vi "UHR-Fleezers Control (fpga) - 11.0.vi"() -> ()   [LabVIEW 2012]
doc: "UHR-Fleezers Instrument Control Code (fpga)"
uses:
  <vilib>/Platform/TimedLoop/XDataNode/timing_clust.ctl
  <vilib>/Platform/TimedLoop/XDataNode/nitl_modes.ctl
  <vilib>/Platform/TimedLoop/XDataNode/wakeup.ctl
  <vilib>/rvi/eio/common/nirviEmuTemplateMethod_errors.vi
  <vilib>/rvi/interface/RandomDataEmulation/nirviRandomDataFPGAFIFO.vi
  <vilib>/rvi/interface/RandomDataEmulation/niFpgaRandomDataHandleErrors.vi
  <vilib>/rvi/Emulation/niFpgaSctlEmulationGetInTimedLoop.vi
  <vilib>/rvi/Emulation/niFpgaSctlEmulationGlobalWrite.vi
  <vilib>/rvi/Emulation/niFpgaSctlEmulationRegisterWithScheduler.vi
  <vilib>/rvi/Emulation/niFpgaSctlEmulationScheduler.vi
  <vilib>/Platform/TimedLoop/XDataNode/XDataNode.xnode
  <vilib>/eio/EIOMethodNode/EIOMethodNode.xnode
  <vilib>/eio/EIONode/EIONode.xnode
  <vilib>/rvi/DataTransferAndStorage/Container/XNode/niFpgaContainer.xnode
  <vilib>/rvi/interface/RandomDataEmulation/nirviRandomDataFpgaReadWriteTemplate.vi
  <vilib>/addons/control/pid/fpga.llb/XNode/niFpgaPID.xnode
  <vilib>/Platform/TimedLoop/XDataNode/XDNodeRunTimeDep.lvlib
panel:
  in  "Connector0/AO6":i16
  in  "Tab Control":T1(tab)=enum."Force FB"
  in  "Trap Pos to FIFO":bool
  in  "AI1 Sets to FIFO":T2={"Set 1"=TRUE, "Set 2"=TRUE, "Set 3"=FALSE}
  in  "N of AI1 Int Acq Sets":i16=2 min=1 max=3 step=1
  out "AI Late Counter":u16
  in  "ai count":u32=400
  out "AI late?":bool
  in  "+ phase":bool
  in  "Phase count adjustment":i16
  out "Relative phase":i16
  in  "AI to FIFO":bool
  out "BD1 Frequency Out 1":u64
  out "BD1 Frequency Out 2":u64
  out "Trap Pos FIFO Timeout":u16
  out "Trap AI FIFO Timeout":u16
  in  "Trap FIFO Set Timeout":i32
  in  "Tab Control 2":T3(tab)
  in  "Swap F1 and F2":bool
  in  "Freq or Amp switch first":bool=TRUE
  in  "Cont. Scan":bool
  in  "Abort scan":bool
  in  "Cycles per step":u64
  in  "Scan BD":bool
  in  "Number of scans":u16
  in  "Scan steps":u64
  in  "Scan freq.  increment":i64
  out "Scanning":bool
  in  "Start scan":bool
  in  "OSK Bd 1":bool
  in  "Reset Bd 1":bool
  in  "RD":bool
  in  "PMODE":bool
  in  "Direct RF Box \nCommunication":bool
  in  "Data BD 2":u8 format="%08b"
  in  "Data BD 1":u8 format="%08b"
  in  "Address":u8 format="%02x"
  in  "Update Data":bool
  in  "FPGA Controls\n RF Box":bool
  in  "Number Interlace Cycles":u8=2 min=1 max=3
  in  "Interlace Off Parameters":u8=1 min=1 max=3
  in  "Interlace ON/OFF":bool
  out "DIO Relative phase":i16
  in  "Phase count adjustment (DIO)":i16
  in  "+ phase (DIO)":bool
  out "DIO Late Counter":u16
  out "DIO Late?":bool
  in  "DIO count 1 (ticks)":u32=400
  in  "DIO count 2 (ticks)":u32=400
  in  "DIO count 3 (ticks)":u32=400
  out "AI2 Y Sum Set 2":i16
  out "AI2 Y Sum Set 1":i16
  in  "FB Gains Set 1":T4={"proportional gain (Kc)"=10, "integral gain (Kc*Ts/Ti)"=5, "derivative gain (Kc*Td/Ts)"=0}
  in  "FB Setpoint Set 1":i16 min=0 step=1
  in  "FB Reset Set 1":bool
  in  "FB On/Off Set 1":bool
  in  "FB Reset Set 2":bool
  in  "FB On/Off Set 2":bool
  in  "FB Setpoint Set 2":i16 min=0 step=1
  in  "FB Gains Set 2":T4={"proportional gain (Kc)"=10, "integral gain (Kc*Ts/Ti)"=5, "derivative gain (Kc*Td/Ts)"=0}
  in  "FB output range 2":cluster{"output high":i16, "output low":i16}={"output high"=3000, "output low"=0}
  in  "FB output range 1":cluster{"output high":i16, "output low":i16}={"output high"=3000, "output low"=0}
  out "Scan I":u64
  in  "Amp switch delay":u16=5
  in  "Freq switch delay":u16
  in  "BD 2 Amplitude 1":u16
  in  "BD 1 Amplitude 1":u16
  in  "BD 2 Frequency 1":u64
  in  "BD 1 Frequency 1":u64
  in  "BD 2 Amplitude 2":u16
  in  "BD 1 Amplitude 2":u16
  in  "BD 2 Frequency 2":u64
  in  "BD 1 Frequency 2":u64
  in  "BD 2 Amplitude 3":u16
  in  "BD 1 Amplitude 3":u16
  in  "BD 2 Frequency 3":u64
  in  "BD 1 Frequency 3":u64
  in  "Negate Diff?":bool
  in  "Diff FB Measurement?":bool
  in  "FB Trig Integrate":u32=1
  out "TTrig?":bool
  in  "TTrig Negate Pos":bool=TRUE
  out "Trap Pos FB Int Signal":fxp<+/-,24,9> format="%.18g"
  out "Trap Pos FB Int-Norm Signal":fxp<+/-,16,1> format="%.16g"
  in  "FPGA TTrig Thresh":i64
  in  "FPGA Trap Trig":bool
  out "Trap Pos FB Action":i64
  in  "Trap Pos. FB Offset Factor":i64
  in  "Trap Pos. FB Mult Factor":i64=2
  in  "Trap Pos. FB Range":T5={"output high"=0.999969482421875, "output low"=-1.0}
  in  "Trap Pos. FB Gains":T6={"proportional gain (Kc)"=0.0, "integral gain (Kc*Ts/Ti)"=10.0, "derivative gain (Kc*Td/Ts)"=0.0} {"proportional gain (Kc)" format="%.11g"; "integral gain (Kc*Ts/Ti)" format="%.11g"; "derivative gain (Kc*Td/Ts)" format="%.11g"}
  in  "Trap Pos. FB Reset":bool
  in  "Trap Pos FB Monitor T1 or T2":bool
  in  "AI1 X Scale":u16
  in  "Trap Pos FB Int Count":u16=100
  in  "Trap Pos FB Negate Action":bool
  out "AI1 X Set 2":fxp<+/-,16,1>
  out "AI1 X Set 1":fxp<+/-,16,1>
  in  "Trap Pos. FB SP":fxp<+/-,16,1>
  in  "Force feedback":bool
  out "TTrig Sig":i64
  out "TTrig Fin Thresh":i64
  out "Numeric":i32
  out "AO2 2":i16
  out "AO1 2":i16
  in  "1D or 2D Scan?":bool
  in  "Abort scan (MCL)":bool
  in  "MCL Scan Axis":bool
  in  "Cont. Scan (MCL)":bool
  out "Scan I (MCL)":u64
  in  "Number of scans (MCL)":u16
  out "Scanning MCL":bool
  in  "Scan steps (MCL)":u64
  in  "Cycles per step (MCL)":u64
  in  "Scan freq.  increment (MCL)":i16
  in  "Start scan (MCL)":bool
  in  "AO2":i16
  in  "AO1":i16
  out "MCL Late Counter":u16
  out "MCL Late?":bool
  in  "MCL count":u32=800
  out "MCL Relative Phase":i16
  in  "Phase count adjustment (MCL)":i16
  in  "+ phase (MCL)":bool
  in  "APD Gate Operating Mode":u8 max=2 step=1
  in  "Invert APD Gate":bool
  in  "APD Gate OFF Count":u32=100
  in  "APD Gate ON Count":u32=300
  out "APD 1 Gate Late Counter":u16
  out "APD 1 Gate Late?":bool
  out "APD 1 Gate Relative Phase":i16
  in  "Phase count adjustment (APD 1 Gate)":i16
  in  "+ phase (APD 1 Gate)":bool
  out "APD 2 Counts 0":u32
  out "APD 2 Counts 1":u32
  out "APD 1 Counts 0":u32
  out "APD 1 Counts 1":u32
  out "APD1 out state":bool
  in  "APD 2 AO scale factor":i16=1
  in  "APD 1 AO scale factor":i16=1
  in  "APD to FIFO":bool
  in  "APD Acq Rate Count":u32=20000000
  out "APD Acq Late Counter":u16
  out "APD Acq Late?":bool
  out "APD Acq Relative Phase":i16
  in  "Phase Count Adjustment (APD Acq)":i16
  in  "+ phase (APD Acq)":bool
  in  "Phase count adjustment (APD 2 Gate)":i16
  out "APD 2 Gate Late Counter":u16
  out "APD 2 Gate Late?":bool
  out "APD 2 Gate Relative Phase":i16
  in  "+ phase (APD 2 Gate)":bool
  out "APD2 out state":bool
  in  "Green Filter Flipper":bool
  in  "Green FB Count":u32=1200
  out "Green Late Counter":u16
  out "Green FB Late?":bool
  out "Green FB Relative Phase":i16
  in  "Phase count adjustment (Green FB)":i16=10
  in  "+ phase (Green FB)":bool
  out "Green FB Sum":i16
  in  "Green int current ON count adj":u32=150
  in  "Current Out":u16=30000
  in  "Green FB On/Off":bool
  in  "Green FB Setpoint":i16=250 min=0 step=1
  in  "Green FB Gains":T4={"proportional gain (Kc)"=10, "integral gain (Kc*Ts/Ti)"=5, "derivative gain (Kc*Td/Ts)"=0}
  in  "Green FB Reset":bool
  in  "Operating Mode 2":u8=2 max=2 step=1
  in  "Invert GI 2":bool
  in  "Green interlace OFF count 2":u32=900
  in  "Green interlace ON count 2":u32=300
  out "GI Late Counter 2":u16
  out "GI Late? 2":bool
  out "GI Relative phase 2":i16
  in  "Phase count adjustment (GI) 2":i16=20
  in  "+ phase (GI) 2":bool
  in  "Green interlace OFF count":u32=100
  out "GI Relative phase":i16
  in  "Phase count adjustment (GI)":i16
  in  "+ phase (GI)":bool
  out "GI Late?":bool
  in  "Green interlace ON count":u32=300
  out "GI Late Counter":u16
  in  "Invert GI":bool
  in  "Operating Mode":u8 max=2 step=1
  in  "+ phase (RI)":bool
  out "RI Relative phase":i16
  out "RI Late?":bool
  out "RI Late Counter":u16
  in  "Red interlace ON count":u32=300
  in  "Red interlace OFF count":u32=100
  in  "Invert RI":bool
  in  "Red Laser Operating Mode":u8 max=2 step=1
  in  "Phase count adjustment (RI)":i16
  out "Red FB Intensity":i16
  in  "Phase count adjustment (Red FB)":i16=10
  in  "Red FB Count":u32=1200
  out "Red Late Counter":u16
  out "Red FB Late?":bool
  out "Red FB Relative Phase":i16
  in  "+ phase (Red FB)":bool
  in  "Chassis2/Mod4/AO1":u16
  # "Only one of these can be on\nat a time:"
  # "Raster Scan AOD"
  # "1 (X)"
  # "2 (Y)"
  # "IR Intensity Feedback (RF BD 1)"
  # "FB Triggering Excitation Laser"
  # "AO1 (Y)"
  # "2D"
  # "1D"
  # "AO2 (X)"
  # "APD AO for aligning"
  # "Detection Loop"
  # "Green fluorescent laser digital gate interlacing loop"
  # "0 Forced ON\n1 Forced OFF\n2 Interlacing"
  # "Red fluorescent laser digital gate interlacing loop"
  # "Detection Loop"
  # "0 Forced ON\n1 Forced OFF\n2 Interlacing"
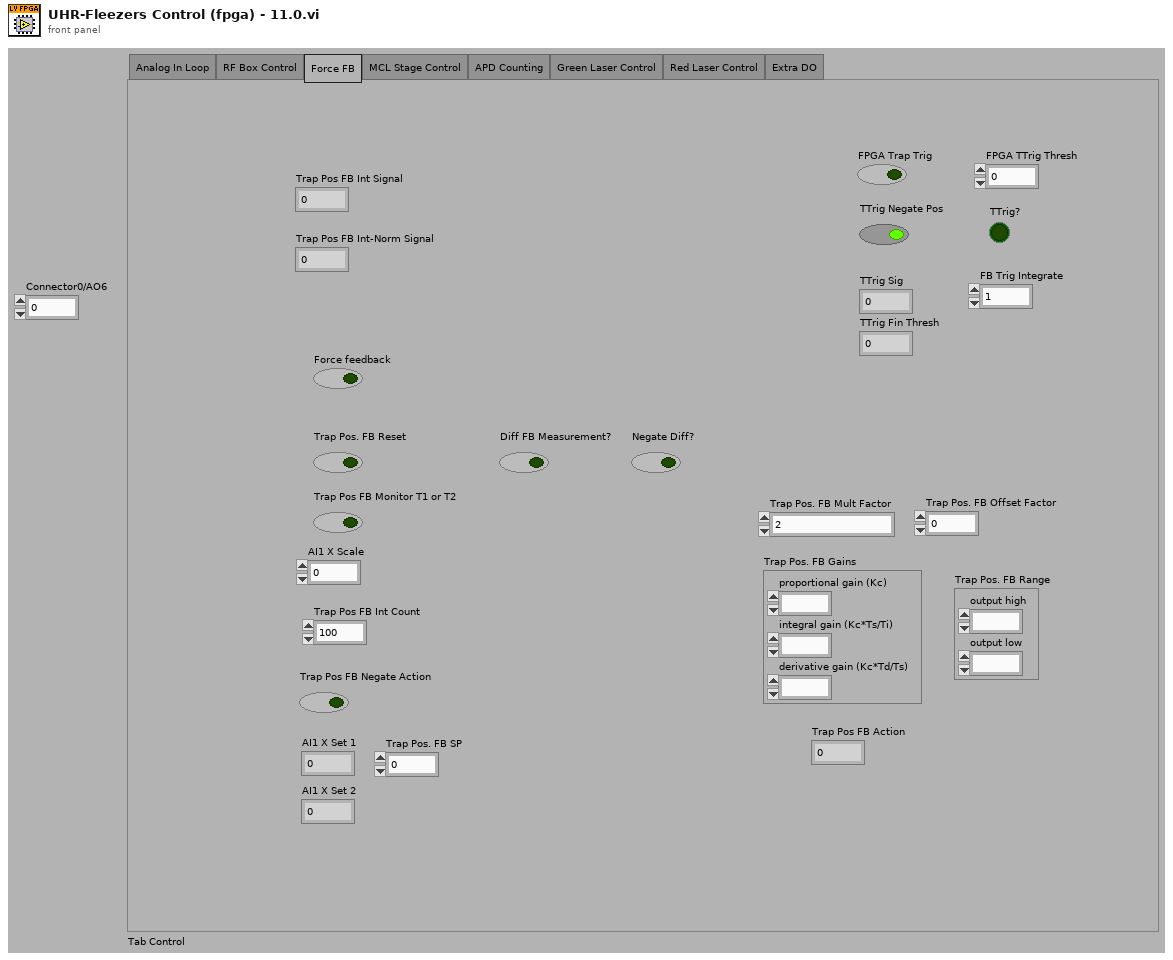
[diagram p1: front panel]
types:
  T1 = enum32{"Analog In Loop", "RF Box Control", "Force FB", "MCL Stage Control", "APD Counting", "Green Laser Control", "Red Laser Control", "Extra DO"}
  T2 = cluster{"Set 1":bool, "Set 2":bool, "Set 3":bool}
  T3 = enum32{"Controls", "Interlacing Frequency and Amplitude Values"}
  T4 = cluster{"proportional gain (Kc)":i16, "integral gain (Kc*Ts/Ti)":i16, "derivative gain (Kc*Td/Ts)":i16}
  T5 = cluster{"output high":fxp<+/-,16,1>, "output low":fxp<+/-,16,1>}
  T6 = cluster{"proportional gain (Kc)":fxp<+/-,16,8>, "integral gain (Kc*Ts/Ti)":fxp<+/-,16,8>, "derivative gain (Kc*Td/Ts)":fxp<+/-,16,8>}
  T7 = typedef "XDNodeRunTimeDep.lvlib/timing_clust.ctl" = cluster{"Expected End [f-1]":u64, "Actual End [f-1]":u64, "Finished Late? [f-1]":bool, "Expected End [i-1]":u64, "Actual End [i-1]":u64, "Finished Late? [i-1]":bool, "Expected Start [i]":u64, "Actual Start [i]":u64, "Expected Start [f]":u64, "Actual Start [f]":u64, "Source Name":string, "Structure Name":string, "Period":i64, "Deadline":i64, "Offset":i64, "Start":i64, "Priority":i32, "Timeout":i32, "Mode":T8, "Wakeup Reason":T9, "Error":errorcluster, "Source Type":string, "Secondary Source Type":string, "Global End Time":u64, "Global Start Time":u64, "Frame Duration":u64, "Iteration Duration":u64, "Assigned CPU":i32, "I/O Scan Engine Mode":u32}
  T8 = typedef "XDNodeRunTimeDep.lvlib/nitl_modes.ctl" = enum32{"No Change", "Process missed periods, maintain original phase", "Discard missed periods, maintain original phase", "Process missed periods, ignore original phase", "Discard missed periods, ignore original phase"}
  T9 = typedef "XDNodeRunTimeDep.lvlib/wakeup.ctl" = enum32{"Normal", "Aborted", "Asynchronous wakeup", "Timing source error", "Timed loop error", "Timeout"}
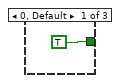
[diagram p2: hidden frame]
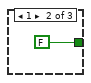
[diagram p3: hidden frame]
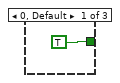
[diagram p4: hidden frame]
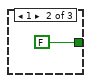
[diagram p5: hidden frame]
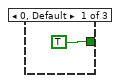
[diagram p7: hidden frame]
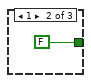
[diagram p8: hidden frame]
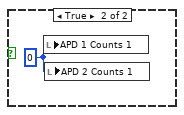
[diagram p9: hidden frame]
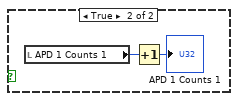
[diagram p11: hidden frame]
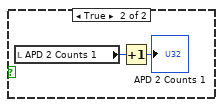
[diagram p12: hidden frame]
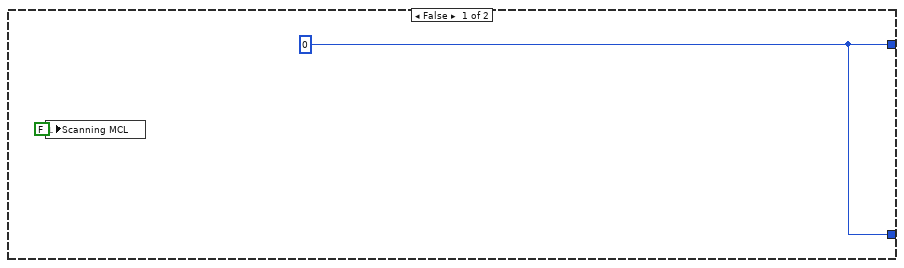
[diagram p13: hidden frame]
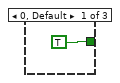
[diagram p14: hidden frame]
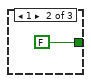
[diagram p15: hidden frame]
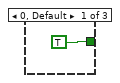
[diagram p16: hidden frame]
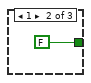
[diagram p17: hidden frame]
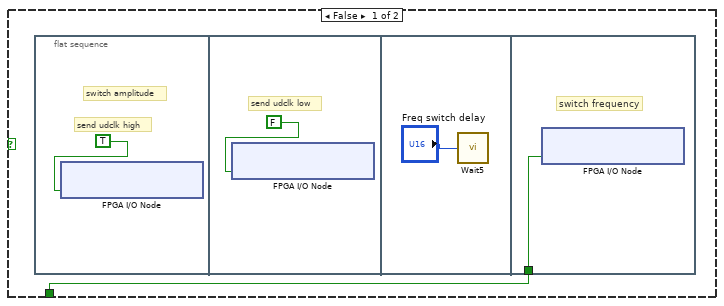
[diagram p20: hidden frame]
diagram:
  w3 = FALSE
  # "timing array current index"
  # "timing array"
  # "timing counter (phase adjusted here)"
  # "late counter"
  n1 = flat-sequence "FPGA initialization to do before running any of the loops" {
    tunnel: [u32 0 ("DIO count 3 (ticks)")] -> w1
    tunnel: [w10] -> _
    frame #0 {
      # "Start up expansion chassis early\nto avoid delays later"
      # "This pin controls udclk on the RF boards.\nWhen initially configuring the boards, this pin needs to be\nconfigured as a high impedance input.  Later it will be switched\nto an output."
      # "Initial setting of DIO data and \naddress to low (before reset).  \nThis needs to happen before the other\ncontrol method loops execute."
      n2 = xnode "FPGA I/O Node"("Chassis2/Mod4/AO0"=u16 0) -> ("Chassis2/Mod1/AI0"=w10:i16)  [unwired: 2 in, 2 out]
      n3 = xnode "FPGA I/O Method Node"("Enable"=FALSE) -> ()  [unwired: 1 in, 1 out]
      n4 = xnode "FPGA I/O Node"("Connector1/DIO0"=FALSE, "Connector1/DIO1"=FALSE, "Connector1/DIO2"=FALSE, "Connector1/DIO3"=FALSE, "Connector1/DIO4"=FALSE, "Connector1/DIO5"=FALSE, "Connector1/DIO6"=FALSE, "Connector1/DIO7"=FALSE, "Connector1/DIO8"=FALSE, "Connector1/DIO9"=FALSE, "Connector1/DIO10"=FALSE, "Connector1/DIO11"=FALSE, "Connector1/DIO12"=FALSE, "Connector1/DIO13"=FALSE, "Connector1/DIO15"=FALSE, "Connector1/DIO20"=FALSE, "Connector1/DIO21"=FALSE, "Connector1/DIO22"=FALSE, "Connector1/DIO23"=FALSE, "Connector1/DIO24"=FALSE, "Connector1/DIO25"=FALSE, "Connector1/DIO26"=FALSE, "Connector1/DIO27"=FALSE, "Connector1/DIO14"=FALSE) -> ()  [unwired: 24 in, 24 out]
    }
  }
  n5 = local read "AO1"() -> (w7:i16)
  n6 = local read "AO2"() -> (w6:i16)
  n7 = node-c288() -> (w5:T7)  [unwired: 1 in]
  n8 = while "APD 1 Counter" {
    tunnel: w1 -> [_]
    stop <- FALSE stop-if-true
    n9 = flat-sequence {
      frame #0 {
        n10 = xnode "FPGA I/O Method Node"("FPGA I/O In"=refnum<k21> "Connector0/DIO0" ("APD 1 DO"), "Timeout"=-1) -> ()  [unwired: 2 out]
      }
      frame #1 {
        n11 = local read "APD1 out state"() -> (w41:bool)
        n12 = case shown="False" w41 {
          frame False {
            n13 = local read "APD 1 Counts 0"() -> (w43:u32)
            n14 = Increment(x=w43) -> (x+1=→"APD 1 Counts 0":u32)
          }
          frame True {
            n15 = local read "APD 1 Counts 1"() -> (w45:u32)
            n16 = Increment(x=w45) -> (x+1=→"APD 1 Counts 1":u32)
          }
        }
      }
    }
  }
  n17 = while "APD 2 Counter" {
    tunnel: w1 -> [_]
    stop <- FALSE stop-if-true
    n18 = flat-sequence {
      frame #0 {
        n19 = xnode "FPGA I/O Method Node"("FPGA I/O In"=refnum<k21> "Connector0/DIO1" ("APD 2 DO"), "Timeout"=-1) -> ()  [unwired: 2 out]
      }
      frame #1 {
        n20 = local read "APD2 out state"() -> (w49:bool)
        n21 = case shown="False" w49 {
          frame False {
            n22 = local read "APD 2 Counts 0"() -> (w51:u32)
            n23 = Increment(x=w51) -> (x+1=→"APD 2 Counts 0":u32)
          }
          frame True {
            n24 = local read "APD 2 Counts 1"() -> (w53:u32)
            n25 = Increment(x=w53) -> (x+1=→"APD 2 Counts 1":u32)
          }
        }
      }
    }
  }
  n26 = while "APD 2 Gating" {
    shift-right: [w57] -> _
    shift-left: w1 -> [w62]
    shift-right: [w56] -> _
    shift-left: w3 -> [w54]
    stop <- FALSE stop-if-true
    n27 = flat-sequence {
      tunnel: w62 -> [w65]
      tunnel: [w66] -> w60
      tunnel: [w65] -> w58
      tunnel: [w64] -> w55
      tunnel: w54 -> [w64]
      tunnel: [w69] -> w61
      tunnel: w60 -> [w69]
      tunnel: [w68] -> w59
      tunnel: w58 -> [w68]
      tunnel: w55 -> [w67]
      tunnel: [w87] -> w57
      tunnel: w61 -> [w98]
      tunnel: w59 -> [w96]
      tunnel: [w91] -> w56
      frame #0 {
        n28 = call "Loop Timer8"("Count(Ticks)"=w65) -> ("Tick Count(Ticks)"=w66:u32)
      }
      frame #1 {
        # "(need 4 channels/APD)"
        n29 = xnode "FPGA I/O Node"("Connector0/DIO8"=w67, "Connector0/DIO9"=w67, "Connector0/DIO10"=w67, "Connector0/DIO11"=w67) -> ()  [unwired: 4 in, 4 out]
      }
      frame #2 {
        n30 = local read "APD Gate ON Count"() -> (w80:u32)
        n31 = local read "APD Gate OFF Count"() -> (w79:u32)
        n32 = feedback #1(TRUE) -> (w93:bool)
        n33 = feedback-in #2(w98) -> ()
        n34 = feedback #2(w98) -> (w81:u32)
        n35 = Not(x=w93) -> (.not. x?=w90:bool)
        n36 = feedback-in #1(w90) -> ()
        n37 = Subtract(x=w98, y=w81) -> (x-y=w97:u32)
        n38 = Select(t=w80, s=w90, f=w79) -> (s? t:f=w95:u32)
        n39 = Subtract(x=w97, y=w96) -> (x-y=w72:u32)
        n40 = Subtract(x=w95, y=w72) -> (x-y=w86:u32)
        n41 = Number To Boolean Array(number=w72) -> (Boolean array=w71:bool[])
        n42 = Or Array Elements(Boolean array=w71) -> (logical OR=w70:bool)
        "APD 2 Gate Late?" <- w70
        n43 = Boolean To (0,1)(Boolean="+ phase (APD 2 Gate)") -> (0, 1=w84:i16)
        n44 = Multiply(x=w84, y="Phase count adjustment (APD 2 Gate)") -> (x*y=w82:i16)
        n45 = Boolean To (0,1)(Boolean=w70) -> (0, 1=w77:i16)
        n46 = Add(x=w86, y=w82) -> (x+y=w87:u32)
        n47 = To Unsigned Word Integer(number=w77) -> (unsigned 16bit integer=w74:u16)
        n48 = feedback #3(i16 0) -> (w89:i16)
        n49 = Subtract(x=w89, y=w82) -> (x-y=w88:i16)
        "APD 2 Gate Relative Phase" <- w88
        n50 = feedback-in #3(w88) -> ()
        n51 = feedback #4(u16 0) -> (w75:u16)
        n52 = Add(x=w74, y=w75) -> (x+y=w73:u16)
        "APD 2 Gate Late Counter" <- w73
        n53 = feedback-in #4(w73) -> ()
        n54 = local read "APD Gate Operating Mode"() -> (w78:u8)
        n55 = case shown="2" w78 {
          tunnel: [TRUE FALSE w104] -> w91
          tunnel: w93 -> [_ _ w102]
          frame 0, Default {
          }
          frame 1 {
          }
          frame 2 {
            n56 = local read "Invert APD Gate"() -> (w101:bool)
            n57 = Not(x=w102) -> (.not. x?=w103:bool)
            n58 = Select(t=w103, s=w101, f=w102) -> (s? t:f=w104:bool)
          }
        }
      }
    }
  }
  n59 = while "DAQ AI set 1" {
    shift-right: [w105] -> _
    shift-left: w1 -> [w110]
    stop <- FALSE stop-if-true
    n60 = flat-sequence {
      tunnel: w110 -> [w120]
      tunnel: [w121] -> w108
      tunnel: [w120] -> w107
      tunnel: [w131] -> w118
      tunnel: [w130] -> w117
      tunnel: [w129] -> w116
      tunnel: [w128] -> w115
      tunnel: [w127] -> w114
      tunnel: [w126] -> w113
      tunnel: [w125] -> w112
      tunnel: [w124] -> w111
      tunnel: [w123] -> w109
      tunnel: w108 -> [w123]
      tunnel: w107 -> [w122]
      tunnel: [w122] -> w106
      tunnel: [w160] -> w105
      tunnel: w118 -> [w188]
      tunnel: w117 -> [w152]
      tunnel: w116 -> [w153]
      tunnel: w115 -> [w187]
      tunnel: w114 -> [w176]
      tunnel: w113 -> [w175]
      tunnel: w112 -> [w174]
      tunnel: w111 -> [w173]
      tunnel: w109 -> [w170]
      tunnel: w106 -> [w167]
      frame #0 {
        n61 = call "Loop Timer3"("Count(Ticks)"=w120) -> ("Tick Count(Ticks)"=w121:u32)
      }
      frame #1 {
        n62 = xnode "FPGA I/O Node"("Connector1/DIO31"=TRUE ("Connector1/DIO33")) -> ("Connector0/AI0"=w131:i16, "Connector0/AI1"=w130:i16, "Connector0/AI2"=w129:i16, "Connector0/AI3"=w128:i16, "Connector0/AI4"=w127:i16, "Connector0/AI5"=w126:i16, "Connector0/AI6"=w125:i16, "Connector0/AI7"=w124:i16)  [unwired: 9 in, 9 out]
      }
      frame #2 {
        w156 = FALSE ("AI to FIFO")
        # "Adjust phase after data acquired if button pressed"
        n63 = feedback #5(i16 1) -> (w180:i16)
        n64 = Increment(x=w180) -> (x+1=w186:i16)
        n65 = Scale By Power Of 2(n="AI1 X Scale", x=w152) -> (x*2^n=w150:i16)
        n66 = Greater?(x=w186, y="N of AI1 Int Acq Sets") -> (0:w183:bool)
        n67 = Select(t=i16 1, s=w183, f=w186) -> (s? t:f=w185:i16)
        n68 = feedback-in #5(w185) -> ()
        n69 = Divide(x=w150, y=w153) -> (x/y=w149:fxp<+/-,16,1>)
        n70 = feedback #6(w156) -> (w154:bool)
        n71 = feedback #7(w156) -> (w172:bool)
        n72 = case shown="1, Default" w180 {
          tunnel: w153 -> [w210 w218 _]
          tunnel: "AI1 Sets to FIFO" -> [w214 w222 w228]
          tunnel: [w213 w221 w227] -> w177
          tunnel: ["AI to FIFO" w220 w226] -> w171
          tunnel: w172 -> [_ w220 w226]
          tunnel: ["Trap Pos to FIFO" w219 w225] -> w155
          tunnel: w154 -> [_ w219 w225]
          tunnel: w149 -> [w209 w217 _]
          tunnel: [w208 w215 FALSE] -> w136
          tunnel: [w207 w216 u64 0 ("BD1 Frequency Out 2")] -> w135
          frame 1, Default {
            n73 = Unbundle By Name(w214) -> ("Set 1"=w213:bool)
            n74 = local read "BD1 Frequency Out 1"() -> (w207:u64)
            n75 = Compound Arithmetic op=AND("Trap Pos to FIFO", w213, "AI to FIFO") -> (w208:bool)
            "AI2 Y Sum Set 1" <- w210
            "AI1 X Set 1" <- w209
          }
          frame 2 {
            n76 = Unbundle By Name(w222) -> ("Set 2"=w221:bool)
            n77 = local read "BD1 Frequency Out 2"() -> (w216:u64)
            n78 = Compound Arithmetic op=AND(w219, w221, w220) -> (w215:bool)
            "AI2 Y Sum Set 2" <- w218
            "AI1 X Set 2" <- w217
          }
          frame 3 {
            n79 = Unbundle By Name(w228) -> ("Set 3"=w227:bool)
          }
        }
        n80 = And(x=w177, y=w171) -> (x .and. y?=w179:bool)
        n81 = case shown="True" w179 {
          tunnel: w188 -> [_ w242]
          tunnel: w152 -> [_ w241]
          tunnel: w153 -> [_ w240]
          tunnel: w187 -> [_ w239]
          tunnel: w176 -> [_ w238]
          tunnel: w175 -> [_ w237]
          tunnel: w174 -> [_ w236]
          tunnel: w173 -> [_ w235]
          tunnel: 0 ("DMA buffer timeout") -> [_ w244]
          frame False {
          }
          frame True {
            n82 = Build Array(w242, w241, w240, w239, w238, w237, w236, w235) -> (w243:i16[])
            n83 = for {
              tunnel: w243 -> [w246] mode=indexing
              tunnel: w244 -> [w247]
              tunnel: [w245] -> w233 mode=indexing
              n84 = xnode ("FIFO Write")("Element"=w246, "Timeout"=w247) -> ("Timed Out?"=w245:bool)  [unwired: 1 in, 1 out]
            }
            n85 = Or Array Elements(Boolean array=w233) -> (logical OR=w230:bool)
            n86 = Boolean To (0,1)(Boolean=w230) -> (0, 1=w232:i16)
            n87 = feedback #8(u16 0) -> (w231:u16)
            n88 = Add(x=w232, y=w231) -> (x+y=w229:u16)
            "Trap AI FIFO Timeout" <- w229
            n89 = feedback-in #8(w229) -> ()
          }
        }
        n90 = feedback-in #6(w155) -> ()
        n91 = feedback-in #7(w171) -> ()
        n92 = case shown="True" w136 {
          tunnel: w135 -> [_ w194]
          tunnel: [u8 0 w191] -> w134
          frame False {
          }
          frame True {
            n93 = Split Number(x=w194) -> (hi(x)=w195:u32, lo(x)=w196:u32)
            n94 = Split Number(x=w195) -> (lo(x)=w197:u16)  [unwired: 1 out]
            n95 = Split Number(x=w196) -> (hi(x)=w198:u16, lo(x)=w199:u16)
            n96 = Build Array "BD 1 nu Stack"(w197, w198, w199) -> (w193:u16[])
            n97 = for {
              tunnel: w193 -> [w206] mode=indexing
              shift-right: [w202] -> w191
              shift-left: u8 0 -> [w203]
              n98 = xnode ("FIFO Method Node")("Element"=w206, "Timeout"="Trap FIFO Set Timeout") -> ("Timed Out?"=w205:bool)  [unwired: 1 in, 1 out]
              n99 = Boolean To (0,1)(Boolean=w205) -> (0, 1=w204:i16)
              n100 = To Unsigned Byte Integer(number=w204) -> (unsigned 8bit integer=w201:u8)
              n101 = Add(x=w201, y=w203) -> (x+y=w202:u8)
            }
          }
        }
        n102 = To Unsigned Word Integer(number=w134) -> (unsigned 16bit integer=w133:u16)
        n103 = feedback #9(u16 0) -> (w147:u16)
        n104 = Add(x=w133, y=w147) -> (x+y=w146:u16)
        "Trap Pos FIFO Timeout" <- w146
        n105 = feedback-in #9(w146) -> ()
        n106 = feedback-in #10(w170) -> ()
        n107 = feedback #10(w170) -> (w169:u32)
        n108 = Subtract(x=w170, y=w169) -> (x-y=w168:u32)
        n109 = xnode "FPGA I/O Node"("Connector1/DIO31"=FALSE ("Connector1/DIO34")) -> ()  [unwired: 1 in, 1 out]
        n110 = Subtract(x=w168, y=w167) -> (x-y=w138:u32)
        n111 = Boolean To (0,1)(Boolean="+ phase") -> (0, 1=w163:i16)
        n112 = Multiply(x=w163, y="Phase count adjustment") -> (x*y=w157:i16)
        n113 = Subtract(x="ai count", y=w138) -> (x-y=w161:u32)
        n114 = Number To Boolean Array(number=w138) -> (Boolean array=w139:bool[])
        n115 = feedback #11(i16 0) -> (w159:i16)
        n116 = Add(x=w161, y=w157) -> (x+y=w160:u32)
        n117 = Subtract(x=w159, y=w157) -> (x-y=w158:i16)
        "Relative phase" <- w158
        n118 = feedback-in #11(w158) -> ()
        n119 = Or Array Elements(Boolean array=w139) -> (logical OR=w137:bool)
        "AI late?" <- w137
        n120 = Boolean To (0,1)(Boolean=w137) -> (0, 1=w144:i16)
        n121 = To Unsigned Word Integer(number=w144) -> (unsigned 16bit integer=w141:u16)
        n122 = feedback #12(u16 0) -> (w142:u16)
        n123 = Add(x=w141, y=w142) -> (x+y=w140:u16)
        "AI Late Counter" <- w140
        n124 = feedback-in #12(w140) -> ()
      }
    }
  }
  n125 = while "MCL stage control" {
    shift-right: [w263] -> _
    shift-left: w1 -> [w266]
    shift-right: [w256] -> _
    shift-left: w7 -> [w253]
    shift-right: [w255] -> _
    shift-left: w6 -> [w251]
    i -> [w250]
    stop <- FALSE stop-if-true
    n126 = flat-sequence {
      tunnel: w266 -> [w270]
      tunnel: [w271] -> w262
      tunnel: [w270] -> w260
      tunnel: [w269] -> w254
      tunnel: w253 -> [w269]
      tunnel: [w268] -> w252
      tunnel: w251 -> [w268]
      tunnel: w262 -> [w275]
      tunnel: [w275] -> w261
      tunnel: w260 -> [w274]
      tunnel: [w274] -> w259
      tunnel: w254 -> [w273]
      tunnel: w252 -> [w272]
      tunnel: [w273] -> w249
      tunnel: [w272] -> w248
      tunnel: w261 -> [w285]
      tunnel: w259 -> [w284]
      tunnel: [w285] -> w265
      tunnel: [w284] -> w264
      tunnel: [w283] -> w258
      tunnel: [w282] -> w257
      tunnel: w249 -> [w277]
      tunnel: w248 -> [w276]
      tunnel: [w357] -> w263
      tunnel: w265 -> [w364]
      tunnel: w264 -> [w361]
      tunnel: w258 -> [w359]
      tunnel: w257 -> [w358]
      tunnel: [w359] -> w256
      tunnel: [w358] -> w255
      frame #0 {
        n127 = call "Loop Timer5"("Count(Ticks)"=w270) -> ("Tick Count(Ticks)"=w271:u32)
      }
      frame #1 {
        n128 = xnode "FPGA I/O Node"("Connector0/AO1"=w273, "Connector0/AO2"=w272) -> ()  [unwired: 2 in, 2 out]
      }
      frame #2 {
        n129 = local read "Scanning MCL"() -> (w297:bool)
        n130 = Or(x=w297, y="Start scan (MCL)") -> (x .or. y?=w292:bool)
        n131 = Not(x="Abort scan (MCL)") -> (.not. x?=w290:bool)
        n132 = And(x=w290, y=w292) -> (x .and. y?=w289:bool)
        n133 = case "Raster scan" shown="True" w289 {
          tunnel: [w298 w341] -> w294
          tunnel: "Start scan (MCL)" -> [_ w326]
          tunnel: [w298 w302] -> w278
          frame False {
            w298 = i16 0
            n134 = local write "Scanning MCL"(FALSE ("scanning")) -> ()
          }
          frame True {
            w312 = i16 0
            w311 = u64 0
            # "scan incr."
            # "freq. incr. mult."
            # "count steps"
            # "count number of cycles"
            n135 = feedback #13(w311) -> (w338:u64)
            n136 = Select(t=w311, s=w326, f=w338) -> (s? t:f=w340:u64)
            n137 = Increment(x=w340) -> (x+1=w337:u64)
            n138 = Greater?(x="Cycles per step (MCL)", y=w337) -> (0:w321:bool)
            n139 = Select(t=w337, s=w321, f=w311) -> (s? t:f=w336:u64)
            n140 = feedback-in #13(w336) -> ()
            n141 = feedback #14(w311) -> (w335:u64)
            n142 = Select(t=w311, s=w326, f=w335) -> (s? t:f=w330:u64)
            n143 = Increment(x=w330) -> (x+1=w334:u64)
            n144 = Add(x="Scan steps (MCL)", y="Scan steps (MCL)") -> (x+y=w333:u64)
            n145 = Select(t=w330, s=w321, f=w334) -> (s? t:f=w316:u64)
            n146 = Greater?(x=w333, y=w316) -> (0:w315:bool)
            n147 = Select(t=w316, s=w315, f=w311) -> (s? t:f=w331:u64)
            n148 = feedback-in #14(w331) -> ()
            n149 = Equal?(x="Scan steps (MCL)", y=w316) -> (x = y?=w320:bool)
            n150 = Greater?(x="Scan steps (MCL)", y=w330) -> (0:w329:bool)
            n151 = feedback #15(w312) -> (w332:i16)
            n152 = Select(t=w312, s=w326, f=w332) -> (s? t:f=w318:i16)
            n153 = Increment(x=w318) -> (x+1=w328:i16)
            n154 = Decrement(x=w318) -> (x-1=w327:i16)
            n155 = Select(t=w328, s=w329, f=w327) -> (s? t:f=w319:i16)
            n156 = Select(t=w318, s=w320, f=w319) -> (s? t:f=w317:i16)
            n157 = Select(t=w318, s=w321, f=w317) -> (s? t:f=w313:i16)
            n158 = Select(t=w313, s=w315, f=w312) -> (s? t:f=w314:i16)
            n159 = feedback-in #15(w314) -> ()
            n160 = feedback #16(w311) -> (w325:u64)
            n161 = Select(t=w311, s=w326, f=w325) -> (s? t:f=w300:u64)
            n162 = Increment(x=w300) -> (x+1=w322:u64)
            n163 = Select(t=w300, s=w315, f=w322) -> (s? t:f=w301:u64)
            n164 = Greater?(x="Number of scans (MCL)", y=w301) -> (0:w308:bool)
            n165 = Multiply(x="Scan freq.  increment (MCL)", y=w318) -> (x*y=w341:i16)
            n166 = Select(t=TRUE, s="Cont. Scan (MCL)", f=w308) -> (s? t:f=w307:bool)
            "Scanning MCL" <- w307
            n167 = Select(t=w301, s=w307, f=w311) -> (s? t:f=w323:u64)
            n168 = feedback-in #16(w323) -> ()
            n169 = Increment(x=w301) -> (x+1=→"Scan I (MCL)":u64)
            n170 = To Word Integer(number=w300) -> (16bit integer=w303:i16)
            n171 = Multiply(x=w303, y="Scan freq.  increment (MCL)") -> (x*y=w302:i16)
          }
        }
        n172 = Select(t=w278, s="1D or 2D Scan?", f=i16 0) -> (s? t:f=w279:i16)
        n173 = Select(t=w279, s="MCL Scan Axis", f=w294) -> (s? t:f=w293:i16)
        n174 = Select(t=w294, s="MCL Scan Axis", f=w279) -> (s? t:f=w295:i16)
        n175 = Add(x=w293, y="AO2") -> (x+y=w282:i16)
        n176 = Add(x="AO1", y=w295) -> (x+y=w283:i16)
        "AO1 2" <- w277
        "AO2 2" <- w276
      }
      frame #3 {
        n177 = feedback-in #17(w364) -> ()
        n178 = feedback #17(w364) -> (w363:u32)
        n179 = Boolean To (0,1)(Boolean="+ phase (MCL)") -> (0, 1=w355:i16)
        n180 = Subtract(x=w364, y=w363) -> (x-y=w362:u32)
        n181 = Multiply(x=w355, y="Phase count adjustment (MCL)") -> (x*y=w351:i16)
        n182 = Subtract(x=w362, y=w361) -> (x-y=w343:u32)
        n183 = Subtract(x="MCL count", y=w343) -> (x-y=w353:u32)
        n184 = feedback #18(i16 0) -> (w352:i16)
        n185 = Subtract(x=w352, y=w351) -> (x-y=w350:i16)
        "MCL Relative Phase" <- w350
        n186 = feedback-in #18(w350) -> ()
        n187 = Number To Boolean Array(number=w343) -> (Boolean array=w344:bool[])
        n188 = Or Array Elements(Boolean array=w344) -> (logical OR=w342:bool)
        "MCL Late?" <- w342
        n189 = Boolean To (0,1)(Boolean=w342) -> (0, 1=w349:i16)
        n190 = Add(x=w353, y=w351) -> (x+y=w357:u32)
        n191 = To Unsigned Word Integer(number=w349) -> (unsigned 16bit integer=w346:u16)
        n192 = feedback #19(u16 0) -> (w347:u16)
        n193 = Add(x=w346, y=w347) -> (x+y=w345:u16)
        "MCL Late Counter" <- w345
        n194 = feedback-in #19(w345) -> ()
      }
    }
    "Numeric" <- w250
  }
  n195 = while "APD 1 Gating" {
    shift-right: [w369] -> _
    shift-left: w1 -> [w374]
    shift-right: [w368] -> _
    shift-left: w3 -> [w366]
    stop <- FALSE stop-if-true
    n196 = flat-sequence {
      tunnel: w374 -> [w377]
      tunnel: [w378] -> w372
      tunnel: [w377] -> w370
      tunnel: [w376] -> w367
      tunnel: w366 -> [w376]
      tunnel: [w381] -> w373
      tunnel: w372 -> [w381]
      tunnel: [w380] -> w371
      tunnel: w370 -> [w380]
      tunnel: w367 -> [w379]
      tunnel: [w395] -> w369
      tunnel: w373 -> [w410]
      tunnel: w371 -> [w407]
      tunnel: [w399] -> w368
      frame #0 {
        n197 = call "Loop Timer7"("Count(Ticks)"=w377) -> ("Tick Count(Ticks)"=w378:u32)
      }
      frame #1 {
        # "(need 4 channels/APD)"
        n198 = xnode "FPGA I/O Node"("Connector0/DIO4"=w379, "Connector0/DIO5"=w379, "Connector0/DIO6"=w379, "Connector0/DIO7"=w379) -> ()  [unwired: 4 in, 4 out]
      }
      frame #2 {
        n199 = feedback #20(TRUE) -> (w402:bool)
        n200 = feedback-in #21(w410) -> ()
        n201 = feedback #21(w410) -> (w409:u32)
        n202 = Not(x=w402) -> (.not. x?=w398:bool)
        n203 = feedback-in #20(w398) -> ()
        n204 = Subtract(x=w410, y=w409) -> (x-y=w408:u32)
        n205 = Select(t="APD Gate ON Count", s=w398, f="APD Gate OFF Count") -> (s? t:f=w404:u32)
        n206 = Subtract(x=w408, y=w407) -> (x-y=w383:u32)
        n207 = Subtract(x=w404, y=w383) -> (x-y=w394:u32)
        n208 = Number To Boolean Array(number=w383) -> (Boolean array=w384:bool[])
        n209 = Or Array Elements(Boolean array=w384) -> (logical OR=w382:bool)
        "APD 1 Gate Late?" <- w382
        n210 = Boolean To (0,1)(Boolean="+ phase (APD 1 Gate)") -> (0, 1=w392:i16)
        n211 = Boolean To (0,1)(Boolean=w382) -> (0, 1=w389:i16)
        n212 = Multiply(x=w392, y="Phase count adjustment (APD 1 Gate)") -> (x*y=w390:i16)
        n213 = To Unsigned Word Integer(number=w389) -> (unsigned 16bit integer=w386:u16)
        n214 = Add(x=w394, y=w390) -> (x+y=w395:u32)
        n215 = feedback #22(i16 0) -> (w397:i16)
        n216 = Subtract(x=w397, y=w390) -> (x-y=w396:i16)
        "APD 1 Gate Relative Phase" <- w396
        n217 = feedback-in #22(w396) -> ()
        n218 = feedback #23(u16 0) -> (w387:u16)
        n219 = Add(x=w386, y=w387) -> (x+y=w385:u16)
        "APD 1 Gate Late Counter" <- w385
        n220 = feedback-in #23(w385) -> ()
        n221 = case shown="2" "APD Gate Operating Mode" {
          tunnel: [TRUE FALSE w416] -> w399
          tunnel: w402 -> [_ _ w413]
          frame 0, Default {
          }
          frame 1 {
          }
          frame 2 {
            n222 = Not(x=w413) -> (.not. x?=w415:bool)
            n223 = Select(t=w415, s="Invert APD Gate", f=w413) -> (s? t:f=w416:bool)
          }
        }
      }
    }
  }
  n224 = while "RF box board direct communication loop" {
    tunnel: w1 -> [_]
    stop <- FALSE stop-if-true
    n225 = case "Whether to use direct communication method (only use one method at a time)" shown="True" "Direct RF Box \nCommunication" {
      frame False {
      }
      frame True {
        n226 = case shown="True" "Update Data" {
          frame False {
          }
          frame True {
            n227 = flat-sequence {
              frame #0 {
                n228 = First Call?() -> (First Call?: T/F=w420:bool)
                n229 = case shown="True" w420 {
                  frame False {
                  }
                  frame True {
                    # "If first time data updated, be sure to set WR high\nbefore setting data and address bits."
                    n230 = flat-sequence {
                      frame #0 {
                        n231 = xnode "FPGA I/O Node"("Connector1/DIO15"=TRUE) -> ()  [unwired: 1 in, 1 out]
                      }
                      frame #1 {
                        n232 = call "Wait"("Count(Ticks)"=u8 40 ("DO Delay 3 (Ticks)")) -> ()  [unwired: 1 out]
                      }
                    }
                  }
                }
              }
              frame #1 {
                n233 = Number To Boolean Array(number="Address") -> (Boolean array=w469:bool[])
                n234 = Number To Boolean Array(number="Data BD 1") -> (Boolean array=w470:bool[])
                n235 = Number To Boolean Array(number="Data BD 2") -> (Boolean array=w439:bool[])
                n236 = Index Array(array=w470, index=7) -> (element=w454:bool)
                n237 = Index Array(array=w470, index=6) -> (element=w453:bool)
                n238 = Index Array(array=w470, index=5) -> (element=w452:bool)
                n239 = Index Array(array=w470, index=4) -> (element=w451:bool)
                n240 = Index Array(array=w470, index=3) -> (element=w450:bool)
                n241 = Index Array(array=w470, index=2) -> (element=w449:bool)
                n242 = Index Array(array=w470, index=1) -> (element=w448:bool)
                n243 = Index Array(array=w470, index=0) -> (element=w447:bool)
                n244 = Index Array(array=w469, index=5) -> (element=w446:bool)
                n245 = Index Array(array=w469, index=4) -> (element=w445:bool)
                n246 = Index Array(array=w469, index=3) -> (element=w444:bool)
                n247 = Index Array(array=w469, index=2) -> (element=w443:bool)
                n248 = Index Array(array=w469, index=1) -> (element=w442:bool)
                n249 = Index Array(array=w469, index=0) -> (element=w441:bool)
                n250 = Index Array(array=w439, index=7) -> (element=w430:bool)
                n251 = Index Array(array=w439, index=6) -> (element=w429:bool)
                n252 = Index Array(array=w439, index=5) -> (element=w428:bool)
                n253 = Index Array(array=w439, index=4) -> (element=w427:bool)
                n254 = Index Array(array=w439, index=3) -> (element=w426:bool)
                n255 = Index Array(array=w439, index=2) -> (element=w425:bool)
                n256 = Index Array(array=w439, index=1) -> (element=w424:bool)
                n257 = Index Array(array=w439, index=0) -> (element=w423:bool)
                n258 = xnode "FPGA I/O Node"("Connector1/DIO0"=w454, "Connector1/DIO1"=w453, "Connector1/DIO2"=w452, "Connector1/DIO3"=w451, "Connector1/DIO4"=w450, "Connector1/DIO5"=w449, "Connector1/DIO6"=w448, "Connector1/DIO7"=w447, "Connector1/DIO8"=w446, "Connector1/DIO9"=w445, "Connector1/DIO10"=w444, "Connector1/DIO11"=w443, "Connector1/DIO12"=w442, "Connector1/DIO13"=w441, "Connector1/DIO20"=w430, "Connector1/DIO21"=w429, "Connector1/DIO22"=w428, "Connector1/DIO23"=w427, "Connector1/DIO24"=w426, "Connector1/DIO25"=w425, "Connector1/DIO26"=w424, "Connector1/DIO27"=w423) -> ()  [unwired: 22 in, 22 out]
              }
              frame #2 {
                # "wait and then apply write signal"
                n259 = call "Wait2"("Count(Ticks)"=u8 40 ("DO Delay 1 (Ticks)")) -> ()  [unwired: 1 out]
              }
              frame #3 {
                # "sending bit low writes data to board buffer"
                n260 = xnode "FPGA I/O Node"("Connector1/DIO15"=FALSE) -> ()  [unwired: 1 in, 1 out]
              }
              frame #4 {
                # "wait then return write signal"
                n261 = call "Wait3"("Count(Ticks)"=u8 40 ("DO Delay 2 (Ticks)")) -> ()  [unwired: 1 out]
              }
              frame #5 {
                # "sending bit high makes ready to\nwrite more data"
                n262 = xnode "FPGA I/O Node"("Connector1/DIO15"=TRUE) -> ()  [unwired: 1 in, 1 out]
              }
            }
          }
        }
      }
    }
  }
  n263 = while "Control APD data integration - stream to host" {
    shift-right: [w479] -> _
    shift-left: w1 -> [w484]
    stop <- FALSE stop-if-true
    n264 = flat-sequence {
      tunnel: w484 -> [w486]
      tunnel: [w487] -> w482
      tunnel: [w486] -> w480
      tunnel: [w495] -> w483
      tunnel: w482 -> [w495]
      tunnel: [w494] -> w481
      tunnel: w480 -> [w494]
      tunnel: [w493] -> w478
      tunnel: [w492] -> w477
      tunnel: [w529] -> w479
      tunnel: w483 -> [w541]
      tunnel: w481 -> [w538]
      tunnel: w478 -> [w522]
      tunnel: w477 -> [w521]
      frame #0 {
        n265 = call "Loop Timer6"("Count(Ticks)"=w486) -> ("Tick Count(Ticks)"=w487:u32)
      }
      frame #1 {
        n266 = flat-sequence {
          tunnel: [w497] -> w491
          tunnel: w491 -> [w499]
          tunnel: [w501] -> w490
          tunnel: [w500] -> w489
          tunnel: [w499] -> w488
          tunnel: [w507] -> w492
          tunnel: [w508] -> w493
          tunnel: w490 -> [w508]
          tunnel: w489 -> [w507]
          tunnel: w488 -> [w506]
          frame #0 {
            # "use two separate variable so each APD won't\nhave to wait to read"
            n267 = feedback #24(FALSE) -> (w496:bool)
            "APD1 out state" <- w496
            "APD2 out state" <- w496
            n268 = Not(x=w496) -> (.not. x?=w497:bool)
            n269 = feedback-in #24(w497) -> ()
          }
          frame #1 {
            n270 = local read "APD 1 Counts 1"() -> (w505:u32)
            n271 = local read "APD 1 Counts 0"() -> (w504:u32)
            n272 = local read "APD 2 Counts 1"() -> (w503:u32)
            n273 = local read "APD 2 Counts 0"() -> (w502:u32)
            n274 = Select(t=w505, s=w499, f=w504) -> (s? t:f=w501:u32)
            n275 = Select(t=w503, s=w499, f=w502) -> (s? t:f=w500:u32)
          }
          frame #2 {
            n276 = case shown="False" w506 {
              frame False {
                w509 = u32 0 ("APD 1 Counts 0")
                n277 = local write "APD 1 Counts 0"(w509) -> ()
                n278 = local write "APD 2 Counts 0"(w509) -> ()
              }
              frame True {
                w510 = u32 0 ("APD 1 Counts 1")
                n279 = local write "APD 1 Counts 1"(w510) -> ()
                n280 = local write "APD 2 Counts 1"(w510) -> ()
              }
            }
          }
        }
      }
      frame #2 {
        n281 = feedback-in #25(w541) -> ()
        n282 = feedback #25(w541) -> (w540:u32)
        n283 = Subtract(x=w541, y=w540) -> (x-y=w539:u32)
        n284 = Subtract(x=w539, y=w538) -> (x-y=w514:u32)
        n285 = case shown="True" "APD to FIFO" {
          tunnel: w522 -> [_ w544]
          tunnel: w521 -> [_ w542]
          frame False {
          }
          frame True {
            n286 = flat-sequence {
              tunnel: 0 ("Timeout") -> [w546]
              tunnel: w544 -> [w547]
              tunnel: [w546] -> w543
              tunnel: w543 -> [w549]
              tunnel: w542 -> [w548]
              frame #0 {
                n287 = xnode ("FIFO Write")("Element"=w547, "Timeout"=w546) -> ()  [unwired: 1 in, 2 out]
              }
              frame #1 {
                n288 = xnode ("FIFO Write")("Element"=w548, "Timeout"=w549) -> ()  [unwired: 1 in, 2 out]
              }
            }
          }
        }
        n289 = Subtract(x="APD Acq Rate Count", y=w514) -> (x-y=w530:u32)
        n290 = Number To Boolean Array(number=w514) -> (Boolean array=w515:bool[])
        n291 = Or Array Elements(Boolean array=w515) -> (logical OR=w513:bool)
        "APD Acq Late?" <- w513
        n292 = Boolean To (0,1)(Boolean=w513) -> (0, 1=w520:i16)
        n293 = To Unsigned Word Integer(number=w520) -> (unsigned 16bit integer=w517:u16)
        n294 = Boolean To (0,1)(Boolean="+ phase (APD Acq)") -> (0, 1=w526:i16)
        n295 = feedback #26(u16 0) -> (w518:u16)
        n296 = Add(x=w517, y=w518) -> (x+y=w516:u16)
        "APD Acq Late Counter" <- w516
        n297 = feedback-in #26(w516) -> ()
        n298 = Multiply(x=w526, y="Phase Count Adjustment (APD Acq)") -> (x*y=w523:i16)
        n299 = Add(x=w530, y=w523) -> (x+y=w529:u32)
        n300 = feedback #27(i16 0) -> (w528:i16)
        n301 = Subtract(x=w528, y=w523) -> (x-y=w525:i16)
        "APD Acq Relative Phase" <- w525
        n302 = feedback-in #27(w525) -> ()
        n303 = To Word Integer(number=w522) -> (16bit integer=w531:i16)
        n304 = To Word Integer(number=w521) -> (16bit integer=w532:i16)
        n305 = Multiply(x="APD 1 AO scale factor", y=w531) -> (x*y=w512:i16)
        n306 = Multiply(x="APD 2 AO scale factor", y=w532) -> (x*y=w511:i16)
        n307 = xnode "FPGA I/O Node"("Connector0/AO5"=w512, "Connector0/AO7"=w511) -> ()  [unwired: 2 in, 2 out]
      }
    }
  }
  n308 = timed-loop "RF box board DIO control: control bits" {
    timing: w5 -> [_]
    timing-out: [_] -> w4
    tunnel: [w550] -> _
    tunnel: w1 -> [w550]
    stop <- FALSE stop-if-true
    n309 = xnode "FPGA I/O Node"("Connector1/DIO16"="RD", "Connector1/DIO17"="PMODE", "Connector1/DIO18"="OSK Bd 1", "Connector1/DIO19"="Reset Bd 1") -> ()  [unwired: 4 in, 4 out]
  }
  n310 = while "532 nm green fluorescent laser interlacing (DO to IA 532 nm AOM ME amp)." {
    shift-right: [w561] -> _
    shift-left: w1 -> [w566]
    shift-right: [w560] -> _
    shift-left: FALSE -> [w558]
    stop <- FALSE stop-if-true
    n311 = flat-sequence {
      tunnel: w566 -> [w569]
      tunnel: [w570] -> w564
      tunnel: [w569] -> w562
      tunnel: [w568] -> w559
      tunnel: w558 -> [w568]
      tunnel: [w573] -> w565
      tunnel: w564 -> [w573]
      tunnel: [w572] -> w563
      tunnel: w562 -> [w572]
      tunnel: w559 -> [w571]
      tunnel: [w582] -> w561
      tunnel: w565 -> [w602]
      tunnel: w563 -> [w599]
      tunnel: [w591] -> w560
      frame #0 {
        n312 = call "Loop Timer4"("Count(Ticks)"=w569) -> ("Tick Count(Ticks)"=w570:u32)
      }
      frame #1 {
        n313 = xnode "FPGA I/O Node"("Connector1/DIO37"=w571, "Connector1/DIO38"=w571, "Connector1/DIO39"=w571) -> ()  [unwired: 3 in, 3 out]
      }
      frame #2 {
        n314 = feedback-in #28(w602) -> ()
        n315 = feedback #28(w602) -> (w601:u32)
        n316 = Subtract(x=w602, y=w601) -> (x-y=w600:u32)
        n317 = Subtract(x=w600, y=w599) -> (x-y=w575:u32)
        n318 = Number To Boolean Array(number=w575) -> (Boolean array=w576:bool[])
        n319 = Or Array Elements(Boolean array=w576) -> (logical OR=w574:bool)
        "GI Late?" <- w574
        n320 = Boolean To (0,1)(Boolean="+ phase (GI)") -> (0, 1=w587:i16)
        n321 = Multiply(x=w587, y="Phase count adjustment (GI)") -> (x*y=w584:i16)
        n322 = Boolean To (0,1)(Boolean=w574) -> (0, 1=w581:i16)
        n323 = To Unsigned Word Integer(number=w581) -> (unsigned 16bit integer=w578:u16)
        n324 = feedback #29(i16 0) -> (w585:i16)
        n325 = feedback #30(u16 0) -> (w579:u16)
        n326 = Add(x=w578, y=w579) -> (x+y=w577:u16)
        "GI Late Counter" <- w577
        n327 = feedback-in #30(w577) -> ()
        n328 = Subtract(x=w585, y=w584) -> (x-y=w583:i16)
        "GI Relative phase" <- w583
        n329 = feedback-in #29(w583) -> ()
        n330 = feedback #31(TRUE) -> (w594:bool)
        n331 = case shown="2" "Operating Mode" {
          tunnel: [TRUE FALSE w608] -> w591
          tunnel: w594 -> [_ _ w605]
          frame 0, Default {
          }
          frame 1 {
          }
          frame 2 {
            n332 = Not(x=w605) -> (.not. x?=w607:bool)
            n333 = Select(t=w607, s="Invert GI", f=w605) -> (s? t:f=w608:bool)
          }
        }
        n334 = Not(x=w594) -> (.not. x?=w590:bool)
        n335 = Select(t="Green interlace ON count", s=w590, f="Green interlace OFF count") -> (s? t:f=w596:u32)
        n336 = Subtract(x=w596, y=w575) -> (x-y=w588:u32)
        n337 = Add(x=w588, y=w584) -> (x+y=w582:u32)
        n338 = feedback-in #31(w590) -> ()
      }
    }
  }
  n339 = while "Green fluorescent laser interlacing (Current to IA 532 nm AOM ME amp)." {
    shift-right: [w614] -> _
    shift-left: w1 -> [w617]
    shift-right: [w611] -> _
    shift-left: u16 0 -> [w609]
    stop <- FALSE stop-if-true
    n340 = flat-sequence {
      tunnel: w617 -> [w620]
      tunnel: [w621] -> w616
      tunnel: [w620] -> w615
      tunnel: [w619] -> w610
      tunnel: w609 -> [w619]
      tunnel: [w624] -> w613
      tunnel: w616 -> [w624]
      tunnel: [w623] -> w612
      tunnel: w615 -> [w623]
      tunnel: w610 -> [w622]
      tunnel: [w633] -> w614
      tunnel: [w650] -> w611
      tunnel: w613 -> [w663]
      tunnel: w612 -> [w660]
      frame #0 {
        n341 = call "Loop Timer10"("Count(Ticks)"=w620) -> ("Tick Count(Ticks)"=w621:u32)
      }
      frame #1 {
        n342 = xnode "FPGA I/O Node"("Chassis2/Mod4/AO0"=w622) -> ()  [unwired: 1 in, 1 out]
      }
      frame #2 {
        n343 = Subtract(x="Green interlace OFF count 2", y="Green int current ON count adj") -> (x-y=w642:u32)
        n344 = feedback-in #32(w663) -> ()
        n345 = feedback #32(w663) -> (w662:u32)
        n346 = Add(x="Green int current ON count adj", y="Green interlace ON count 2") -> (x+y=w643:u32)
        n347 = Subtract(x=w663, y=w662) -> (x-y=w661:u32)
        n348 = Subtract(x=w661, y=w660) -> (x-y=w626:u32)
        n349 = Number To Boolean Array(number=w626) -> (Boolean array=w627:bool[])
        n350 = Boolean To (0,1)(Boolean="+ phase (GI) 2") -> (0, 1=w639:i16)
        n351 = Or Array Elements(Boolean array=w627) -> (logical OR=w625:bool)
        "GI Late? 2" <- w625
        n352 = Boolean To (0,1)(Boolean=w625) -> (0, 1=w632:i16)
        n353 = Multiply(x=w639, y="Phase count adjustment (GI) 2") -> (x*y=w635:i16)
        n354 = To Unsigned Word Integer(number=w632) -> (unsigned 16bit integer=w628:u16)
        n355 = feedback #33(u16 0) -> (w630:u16)
        n356 = Add(x=w628, y=w630) -> (x+y=w629:u16)
        "GI Late Counter 2" <- w629
        n357 = feedback-in #33(w629) -> ()
        n358 = feedback #34(i16 0) -> (w636:i16)
        n359 = Subtract(x=w636, y=w635) -> (x-y=w634:i16)
        "GI Relative phase 2" <- w634
        n360 = feedback-in #34(w634) -> ()
        n361 = feedback #35(TRUE) -> (w655:bool)
        n362 = case shown="2" "Operating Mode 2" {
          tunnel: [TRUE FALSE w680] -> w644
          tunnel: w655 -> [_ _ w677]
          frame 0, Default {
          }
          frame 1 {
          }
          frame 2 {
            n363 = Not(x=w677) -> (.not. x?=w679:bool)
            n364 = Select(t=w679, s="Invert GI 2", f=w677) -> (s? t:f=w680:bool)
          }
        }
        n365 = And(x=w644, y="Green FB On/Off") -> (x .and. y?=w645:bool)
        n366 = case shown="True" w645 {
          tunnel: "Current Out" -> [w664 _]
          tunnel: [w664 w669] -> w649
          frame False {
          }
          frame True {
            n367 = local read "Green FB Sum"() -> (w665:i16)
            n368 = call "Slower PID.vi"("process variable"=w665, "reset?"="Green FB Reset", "setpoint"="Green FB Setpoint", "PID gains (x 2^8)"="Green FB Gains", "output range"=cluster{"output high":i16, "output low":i16} {"output high"=32767, "output low"=-32768} ("Green FB output range")) -> ("output"=w673:i16)  [unwired: 10 out]
            n369 = To Long Integer(number=w673) -> (32bit integer=w666:i32)
            n370 = Add(x=w666, y=32768) -> (x+y=w668:i32)
            n371 = To Unsigned Word Integer(number=w668) -> (unsigned 16bit integer=w669:u16)
          }
        }
        n372 = Not(x=w655) -> (.not. x?=w652:bool)
        n373 = Select(t=w643, s=w652, f=w642) -> (s? t:f=w657:u32)
        n374 = Subtract(x=w657, y=w626) -> (x-y=w637:u32)
        n375 = Add(x=w637, y=w635) -> (x+y=w633:u32)
        n376 = feedback-in #35(w652) -> ()
        n377 = Boolean To (0,1)(Boolean=w644) -> (0, 1=w651:i16)
        n378 = To Unsigned Word Integer(number=w651) -> (unsigned 16bit integer=w648:u16)
        n379 = Multiply(x=w648, y=w649) -> (x*y=w650:u16)
      }
    }
  }
  n380 = while "532 nm green excitation laser intensity feedback measurement" {
    shift-right: [w681] -> _
    shift-left: w1 -> [w686]
    stop <- FALSE stop-if-true
    n381 = flat-sequence {
      tunnel: w686 -> [w688]
      tunnel: [w689] -> w684
      tunnel: [w688] -> w682
      tunnel: [w693] -> w685
      tunnel: w684 -> [w693]
      tunnel: [w692] -> w683
      tunnel: w682 -> [w692]
      tunnel: [w705] -> w681
      tunnel: w685 -> [w716]
      tunnel: w683 -> [w713]
      frame #0 {
        n382 = call "Loop Timer9"("Count(Ticks)"=w688) -> ("Tick Count(Ticks)"=w689:u32)
      }
      frame #1 {
        n383 = xnode "FPGA I/O Node"("Connector1/DIO35"=TRUE) -> ("Chassis2/Mod1/AI1"=→"Green FB Sum":i16)  [unwired: 2 in, 2 out]
      }
      frame #2 {
        n384 = feedback-in #36(w716) -> ()
        n385 = feedback #36(w716) -> (w715:u32)
        n386 = Subtract(x=w716, y=w715) -> (x-y=w714:u32)
        n387 = xnode "FPGA I/O Node"("Connector1/DIO35"=FALSE) -> ()  [unwired: 1 in, 1 out]
        n388 = Subtract(x=w714, y=w713) -> (x-y=w695:u32)
        n389 = Subtract(x="Green FB Count", y=w695) -> (x-y=w709:u32)
        n390 = Number To Boolean Array(number=w695) -> (Boolean array=w696:bool[])
        n391 = Or Array Elements(Boolean array=w696) -> (logical OR=w694:bool)
        "Green FB Late?" <- w694
        n392 = Boolean To (0,1)(Boolean="+ phase (Green FB)") -> (0, 1=w707:i16)
        n393 = Boolean To (0,1)(Boolean=w694) -> (0, 1=w701:i16)
        n394 = Multiply(x=w707, y="Phase count adjustment (Green FB)") -> (x*y=w702:i16)
        n395 = Add(x=w709, y=w702) -> (x+y=w705:u32)
        n396 = To Unsigned Word Integer(number=w701) -> (unsigned 16bit integer=w698:u16)
        n397 = feedback #37(i16 0) -> (w704:i16)
        n398 = Subtract(x=w704, y=w702) -> (x-y=w703:i16)
        "Green FB Relative Phase" <- w703
        n399 = feedback-in #37(w703) -> ()
        n400 = feedback #38(u16 0) -> (w699:u16)
        n401 = Add(x=w698, y=w699) -> (x+y=w697:u16)
        "Green Late Counter" <- w697
        n402 = feedback-in #38(w697) -> ()
      }
    }
  }
  n403 = while "Control Additional IO (Green laser flip mount)" {
    stop <- FALSE stop-if-true
    n404 = xnode "FPGA I/O Node"("Connector0/DIO3"="Green Filter Flipper", "Chassis2/Mod4/AO1"="Chassis2/Mod4/AO1", "Connector0/AO6"="Connector0/AO6") -> ()  [unwired: 3 in, 3 out]
    n405 = call "Loop Timer2"("Count(Ticks)"=u32 40000 ("Extra DO Counts")) -> ()  [unwired: 1 out]
  }
  n406 = while "RF box board DIO control: parallel communication" {
    shift-right: [w728] -> _
    shift-left: w1 -> [w727]
    shift-right: [w726] -> _
    shift-left: FALSE ("Swap F1 and F2") -> [w725]
    stop <- FALSE stop-if-true
    n407 = flat-sequence {
      tunnel: w725 -> [w732]
      tunnel: w727 -> [w730]
      tunnel: [w732] -> w724
      tunnel: [w731] -> w723
      tunnel: [w730] -> w722
      tunnel: [w738] -> w728
      tunnel: [w737] -> w726
      tunnel: w724 -> [w736]
      tunnel: w723 -> [w734]
      tunnel: w722 -> [w733]
      frame #0 {
        n408 = call "Loop Timer"("Count(Ticks)"=w730) -> ("Tick Count(Ticks)"=w731:u32)
      }
      frame #1 {
        n409 = flat-sequence {
          tunnel: ["FPGA Controls\n RF Box"] -> w735
          tunnel: w736 -> [w739]
          tunnel: [w779] -> w738
          tunnel: [w792] -> w737
          tunnel: w735 -> [w791]
          tunnel: w734 -> [w785]
          tunnel: w733 -> [w782]
          frame #0 {
            n410 = case shown="True" "FPGA Controls\n RF Box" {
              tunnel: w739 -> [_ w741]
              frame False {
              }
              frame True {
                n411 = flat-sequence {
                  tunnel: w741 -> [w747]
                  frame #0 {
                    n412 = First Call?() -> (First Call?: T/F=w742:bool)
                    n413 = case shown="True" w742 {
                      frame False {
                      }
                      frame True {
                        # "If first time data updated, be sure to set WR high and UDCLK low\nbefore setting data and address bits."
                        n414 = xnode "FPGA I/O Method Node"("Enable"=TRUE) -> ("FPGA I/O Out"=w744:refnum<k21>)  [unwired: 1 in]
                        n415 = xnode "FPGA I/O Node"("Connector1/DIO15"=TRUE) -> ()  [unwired: 1 in, 1 out]
                        n416 = xnode "FPGA I/O Node"("I/O Item"=FALSE ("Connector1/DIO30"), "FPGA I/O In"=w744) -> ()  [unwired: 1 out]
                      }
                    }
                  }
                  frame #1 {
                    n417 = case shown="True" "Freq or Amp switch first" {
                      tunnel: w747 -> [w749 w754]
                      frame False {
                        n418 = flat-sequence {
                          tunnel: w749 -> [w753]
                          frame #0 {
                            # "switch amplitude"
                            # "send udclk high"
                            n419 = xnode "FPGA I/O Node"("Connector1/DIO30"=TRUE ("Connector1/DIO15")) -> ()  [unwired: 1 in, 1 out]
                          }
                          frame #1 {
                            # "send udclk low"
                            n420 = xnode "FPGA I/O Node"("Connector1/DIO30"=FALSE ("Connector1/DIO15")) -> ()  [unwired: 1 in, 1 out]
                          }
                          frame #2 {
                            n421 = call "Wait5"("Count(Ticks)"="Freq switch delay") -> ()  [unwired: 1 out]
                          }
                          frame #3 {
                            # "switch frequency"
                            n422 = xnode "FPGA I/O Node"("Connector1/DIO36"=w753) -> ()  [unwired: 1 in, 1 out]
                          }
                        }
                      }
                      frame True {
                        n423 = flat-sequence {
                          tunnel: w754 -> [w755]
                          frame #0 {
                            # "switch frequency"
                            n424 = xnode "FPGA I/O Node"("Connector1/DIO36"=w755) -> ()  [unwired: 1 in, 1 out]
                          }
                          frame #1 {
                            n425 = call "Wait4"("Count(Ticks)"="Amp switch delay") -> ()  [unwired: 1 out]
                          }
                          frame #2 {
                            # "switch amplitude"
                            # "send udclk high"
                            n426 = xnode "FPGA I/O Node"("Connector1/DIO30"=TRUE ("Connector1/DIO15")) -> ()  [unwired: 1 in, 1 out]
                          }
                          frame #3 {
                            # "send udclk low"
                            n427 = xnode "FPGA I/O Node"("Connector1/DIO30"=FALSE ("Connector1/DIO15")) -> ()  [unwired: 1 in, 1 out]
                          }
                        }
                      }
                    }
                  }
                }
              }
            }
          }
          frame #1 {
            # "This is the prior cycle's on time"
            # "increment timing\nindex, reset to 0 if \nend of matrix"
            # "Reset to begginning (1) when number of cycles reached."
            # "timing index"
            # "build byte stacks for writing data\n(must correspond to addresses array constant)"
            # "Timing housekeeping"
            # "Adjust phase if late\n(maintains constant phase relationship between cycles)"
            n428 = feedback #39(u8 0 ("t")) -> (w788:u8)
            n429 = Increment(x=w788) -> (x+1=w832:u8)
            n430 = Increment(x="Number Interlace Cycles") -> (x+1=w827:u8)
            n431 = Equal?(x=w832, y=w827) -> (x = y?=w834:bool)
            n432 = Select(t=u8 1, s=w834, f=w832) -> (s? t:f=w787:u8)
            n433 = feedback-in #39(w787) -> ()
            n434 = Increment(x=w787) -> (x+1=w829:u8)
            n435 = Equal?(x=w829, y=w827) -> (x = y?=w830:bool)
            n436 = Select(t=u8 1, s=w830, f=w829) -> (s? t:f=w826:u8)
            n437 = Select(t=w826, s="Interlace ON/OFF", f="Interlace Off Parameters") -> (s? t:f=w810:u8)
            n438 = case shown="1, Default" w810 {
              tunnel: [w904 "BD 1 Frequency 2" "BD 1 Frequency 3"] -> w822
              tunnel: [w903 "BD 2 Frequency 2" "BD 2 Frequency 3"] -> w811
              tunnel: ["BD 2 Amplitude 1" "BD 2 Amplitude 2" "BD 2 Amplitude 3"] -> w767
              tunnel: [w892 w1056 "BD 1 Amplitude 3"] -> w770
              frame 1, Default {
                w883 = fxp<+/-,24,9> 0.0 ("AI1 X Set 2")
                w876 = u16 0
                w899 = u64 0 ("f")
                # "This signal integration happens no matter what\nso that correct setpoints can be chosen before \nturning on the FB."
                # "Trap 1"
                n439 = local read "AI1 X Set 2"() -> (w879:fxp<+/-,16,1>)
                n440 = local read "AI1 X Set 1"() -> (w880:fxp<+/-,16,1>)
                n441 = local read "Scanning"() -> (w905:bool)
                n442 = Or(x=w905, y="Start scan") -> (x .or. y?=w897:bool)
                n443 = case shown="False" "Diff FB Measurement?" {
                  tunnel: w879 -> [w913 w922]
                  tunnel: w880 -> [w912 w923]
                  tunnel: [w910 w914] -> w881
                  frame False {
                    n444 = Select(t=w912, s="Trap Pos FB Monitor T1 or T2", f=w913) -> (s? t:f=w910:fxp<+/-,16,1>)
                  }
                  frame True {
                    n445 = Subtract(x=w923, y=w922) -> (x-y=w915:fxp<+/-,17,2>)
                    n446 = Not(x="Negate Diff?") -> (.not. x?=w921:bool)
                    n447 = Boolean To (0,1)(Boolean="Negate Diff?") -> (0, 1=w919:i16)
                    n448 = Boolean To (0,1)(Boolean=w921) -> (0, 1=w920:i16)
                    n449 = Negate(x=w919) -> (-x=w918:i16)
                    n450 = Add(x=w918, y=w920) -> (x+y=w916:i16)
                    n451 = Multiply(x=w916, y=w915) -> (x*y=w914:fxp<+/-,32,17>)
                  }
                }
                n452 = Not(x="Abort scan") -> (.not. x?=w895:bool)
                n453 = And(x=w895, y=w897) -> (x .and. y?=w894:bool)
                n454 = case "For raster scanning" shown="False" w894 {
                  tunnel: [u64 0 w1044] -> w900
                  tunnel: "Start scan" -> [_ w1029]
                  frame False {
                    n455 = local write "Scanning"(FALSE ("scanning")) -> ()
                  }
                  frame True {
                    w1013 = i64 0
                    w1012 = u64 0
                    # "scan incr."
                    # "freq. incr. mult."
                    # "count steps"
                    # "count number of cycles"
                    n456 = feedback #40(w1012) -> (w1041:u64)
                    n457 = Select(t=w1012, s=w1029, f=w1041) -> (s? t:f=w1043:u64)
                    n458 = Increment(x=w1043) -> (x+1=w1040:u64)
                    n459 = Greater?(x="Cycles per step", y=w1040) -> (0:w1022:bool)
                    n460 = Select(t=w1040, s=w1022, f=w1012) -> (s? t:f=w1039:u64)
                    n461 = feedback-in #40(w1039) -> ()
                    n462 = feedback #41(w1012) -> (w1038:u64)
                    n463 = Select(t=w1012, s=w1029, f=w1038) -> (s? t:f=w1033:u64)
                    n464 = Increment(x=w1033) -> (x+1=w1037:u64)
                    n465 = Add(x="Scan steps", y="Scan steps") -> (x+y=w1036:u64)
                    n466 = Select(t=w1033, s=w1022, f=w1037) -> (s? t:f=w1017:u64)
                    n467 = Greater?(x=w1036, y=w1017) -> (0:w1016:bool)
                    n468 = Select(t=w1017, s=w1016, f=w1012) -> (s? t:f=w1034:u64)
                    n469 = feedback-in #41(w1034) -> ()
                    n470 = Equal?(x="Scan steps", y=w1017) -> (x = y?=w1021:bool)
                    n471 = Greater?(x="Scan steps", y=w1033) -> (0:w1032:bool)
                    n472 = feedback #42(w1013) -> (w1035:i64)
                    n473 = Select(t=w1013, s=w1029, f=w1035) -> (s? t:f=w1019:i64)
                    n474 = Increment(x=w1019) -> (x+1=w1031:i64)
                    n475 = Decrement(x=w1019) -> (x-1=w1030:i64)
                    n476 = Select(t=w1031, s=w1032, f=w1030) -> (s? t:f=w1020:i64)
                    n477 = Select(t=w1019, s=w1021, f=w1020) -> (s? t:f=w1018:i64)
                    n478 = Select(t=w1019, s=w1022, f=w1018) -> (s? t:f=w1014:i64)
                    n479 = Select(t=w1014, s=w1016, f=w1013) -> (s? t:f=w1015:i64)
                    n480 = feedback-in #42(w1015) -> ()
                    n481 = feedback #43(w1012) -> (w1028:u64)
                    n482 = Select(t=w1012, s=w1029, f=w1028) -> (s? t:f=w1024:u64)
                    n483 = Increment(x=w1024) -> (x+1=w1025:u64)
                    n484 = Select(t=w1024, s=w1016, f=w1025) -> (s? t:f=w1023:u64)
                    n485 = Greater?(x="Number of scans", y=w1023) -> (0:w1009:bool)
                    n486 = Multiply(x="Scan freq.  increment", y=w1019) -> (x*y=w1044:i64)
                    n487 = Select(t=TRUE, s="Cont. Scan", f=w1009) -> (s? t:f=w1008:bool)
                    "Scanning" <- w1008
                    n488 = Select(t=w1023, s=w1008, f=w1012) -> (s? t:f=w1026:u64)
                    n489 = feedback-in #43(w1026) -> ()
                    n490 = Increment(x=w1023) -> (x+1=→"Scan I":u64)
                  }
                }
                n491 = feedback #44(w876) -> (w875:u16)
                n492 = Increment(x=w875) -> (x+1=w877:u16)
                n493 = Greater Or Equal?(x=w877, y="Trap Pos FB Int Count") -> (x >= y?=w868:bool)
                n494 = Select(t=w876, s=w868, f=w877) -> (s? t:f=w878:u16)
                n495 = feedback-in #44(w878) -> ()
                n496 = feedback #45(w883) -> (w882:fxp<+/-,24,9>)
                n497 = Add(x=w881, y=w882) -> (x+y=w874:fxp<+/-,24,9>)
                n498 = Select(t=w883, s=w868, f=w874) -> (s? t:f=w886:fxp<+/-,24,9>)
                n499 = feedback-in #45(w886) -> ()
                n500 = Divide(x=w874, y="Trap Pos FB Int Count") -> (x/y=w869:fxp<+/-,16,1>)
                n501 = feedback #46(fxp<+/-,24,9> 0.0 ("AI1 X Set 2")) -> (w887:fxp<+/-,24,9>)
                n502 = Select(t=w874, s=w868, f=w887) -> (s? t:f=w888:fxp<+/-,24,9>)
                "Trap Pos FB Int Signal" <- w888
                n503 = feedback-in #46(w888) -> ()
                n504 = feedback #47(fxp<+/-,16,1> 0.0 ("Trap Pos FB Int-Norm Signal")) -> (w871:fxp<+/-,16,1>)
                n505 = Select(t=w869, s=w868, f=w871) -> (s? t:f=w870:fxp<+/-,16,1>)
                "Trap Pos FB Int-Norm Signal" <- w870
                n506 = feedback-in #47(w870) -> ()
                n507 = case "For intensity feedback" shown="True" "FB On/Off Set 1" {
                  tunnel: "BD 1 Amplitude 1" -> [w1046 _]
                  tunnel: [w1046 w1047] -> w892
                  frame False {
                  }
                  frame True {
                    n508 = local read "AI2 Y Sum Set 1"() -> (w1049:i16)
                    n509 = call "Slower PID.vi"("process variable"=w1049, "reset?"="FB Reset Set 1", "setpoint"="FB Setpoint Set 1", "PID gains (x 2^8)"="FB Gains Set 1", "output range"="FB output range 1") -> ("output"=w1052:i16)  [unwired: 10 out]
                    n510 = To Unsigned Word Integer(number=w1052) -> (unsigned 16bit integer=w1047:u16)
                  }
                }
                n511 = case "For position feedback" shown="True" "Force feedback" {
                  tunnel: [i64 0 w929] -> w889
                  tunnel: w869 -> [_ w926]
                  tunnel: w868 -> [_ w925]
                  frame False {
                  }
                  frame True {
                    n512 = feedback #48(i64 0) -> (w928:i64)
                    n513 = case shown="True" w925 {
                      tunnel: [w930 w937] -> w929
                      tunnel: w928 -> [w930 _]
                      tunnel: w926 -> [_ w931]
                      frame False {
                      }
                      frame True {
                        w941 = u32 0
                        n514 = xnode ("PID")("process variable"=w931, "reset?"="Trap Pos. FB Reset", "setpoint"="Trap Pos. FB SP", "PID gains"="Trap Pos. FB Gains", "output range"="Trap Pos. FB Range") -> ("output"=w953:fxp<+/-,16,1>)
                        n515 = Negate(x=w953) -> (-x=w952:fxp<+/-,17,2>)
                        n516 = Select(t=w952, s="Trap Pos FB Negate Action", f=w953) -> (s? t:f=w949:fxp<+/-,17,2>)
                        n517 = Scale By Power Of 2(n=u32 15, x=u32 1) -> (x*2^n=w946:u32)
                        n518 = Multiply(x=w949, y=w946) -> (x*y=w945:fxp<+/-,17,17>)
                        n519 = To Quad Integer(1:w945) -> (0:w957:i64)
                        "Trap Pos FB Action" <- w957
                        n520 = Multiply(x=w957, y="Trap Pos. FB Mult Factor") -> (x*y=w955:i64)
                        n521 = Add(x=w955, y="Trap Pos. FB Offset Factor") -> (x+y=w937:i64)
                        n522 = feedback #49() -> (w938:i64)  [unwired: 1 in]
                        n523 = Add(x=w937, y=w938) -> (x+y=w935:i64)
                        n524 = feedback #50(w941) -> (w943:u32)
                        n525 = Increment(x=w943) -> (x+1=w932:u32)
                        n526 = Greater Or Equal?(x=w932, y="FB Trig Integrate") -> (x >= y?=w933:bool)
                        n527 = Select(t=i64 0, s=w933, f=w935) -> (s? t:f=w939:i64)
                        n528 = feedback-in #49(w939) -> ()
                        n529 = Select(t=w941, s=w933, f=w932) -> (s? t:f=w942:u32)
                        n530 = feedback-in #50(w942) -> ()
                        n531 = And(x=w933, y="FPGA Trap Trig") -> (x .and. y?=w940:bool)
                        n532 = case "Trap FB trigger excitation laser ON" shown="True" w940 {
                          tunnel: w935 -> [_ w963]
                          tunnel: w932 -> [_ w961]
                          frame False {
                          }
                          frame True {
                            n533 = Not(x="TTrig Negate Pos") -> (.not. x?=w970:bool)
                            n534 = Boolean To (0,1)(Boolean="TTrig Negate Pos") -> (0, 1=w968:i16)
                            n535 = Boolean To (0,1)(Boolean=w970) -> (0, 1=w969:i16)
                            n536 = Negate(x=w968) -> (-x=w967:i16)
                            n537 = Add(x=w967, y=w969) -> (x+y=w966:i16)
                            n538 = Multiply(x=w966, y=w963) -> (x*y=w965:i64)
                            "TTrig Sig" <- w965
                            n539 = Multiply(x="FPGA TTrig Thresh", y=w961) -> (x*y=w962:i64)
                            "TTrig Fin Thresh" <- w962
                            n540 = Greater Or Equal?(x=w965, y=w962) -> (x >= y?=w964:bool)
                            n541 = case shown="True" w964 {
                              frame False {
                              }
                              frame True {
                                w973 = TRUE ("Green FB On/Off")
                                w975 = u8 2 ("Operating Mode")
                                n542 = local write "Operating Mode 2"(w975) -> ()
                                n543 = local write "Operating Mode"(w975) -> ()
                                n544 = local write "Green FB On/Off"(w973) -> ()
                                n545 = local write "FPGA Trap Trig"(FALSE ("FPGA Trap Trig")) -> ()
                                "TTrig?" <- w973
                              }
                            }
                          }
                        }
                      }
                    }
                    n546 = feedback-in #48(w929) -> ()
                  }
                }
                n547 = Select(t=w899, s="Scan BD", f=w900) -> (s? t:f=w898:u64)
                n548 = Select(t=w900, s="Scan BD", f=w899) -> (s? t:f=w901:u64)
                n549 = Add(x=w898, y="BD 2 Frequency 1") -> (x+y=w903:u64)
                n550 = Compound Arithmetic op=ADD("BD 1 Frequency 1", w889, w901) -> (w904:u64)
                "BD1 Frequency Out 1" <- w904
              }
              frame 2 {
                # "Trap 2"
                n551 = case shown="True" "FB On/Off Set 2" {
                  tunnel: [w1060 w1061] -> w1056
                  tunnel: "BD 1 Amplitude 2" -> [w1060 _]
                  frame False {
                  }
                  frame True {
                    n552 = local read "AI2 Y Sum Set 2"() -> (w1066:i16)
                    n553 = call "Slower PID.vi"("process variable"=w1066, "reset?"="FB Reset Set 2", "setpoint"="FB Setpoint Set 2", "PID gains (x 2^8)"="FB Gains Set 2", "output range"="FB output range 2") -> ("output"=w1063:i16)  [unwired: 10 out]
                    n554 = To Unsigned Word Integer(number=w1063) -> (unsigned 16bit integer=w1061:u16)
                  }
                }
                "BD1 Frequency Out 2" <- "BD 1 Frequency 2"
              }
              frame 3 {
                # "Fluorescence period"
              }
            }
            n555 = feedback-in #51(w785) -> ()
            n556 = feedback #51(w785) -> (w784:u32)
            n557 = Select(t=w787, s="Interlace ON/OFF", f="Interlace Off Parameters") -> (s? t:f=w825:u8)
            n558 = Subtract(x=w785, y=w784) -> (x-y=w783:u32)
            n559 = Subtract "The error"(x=w783, y=w782) -> (x-y=w760:u32)
            n560 = case shown="1, Default" w825 {
              tunnel: ["DIO count 1 (ticks)" "DIO count 2 (ticks)" "DIO count 3 (ticks)"] -> w781
              frame 1, Default {
              }
              frame 2 {
              }
              frame 3 {
              }
            }
            n561 = Number To Boolean Array(number=w760) -> (Boolean array=w761:bool[])
            n562 = Or Array Elements(Boolean array=w761) -> (logical OR=w759:bool)
            "DIO Late?" <- w759
            n563 = Boolean To (0,1)(Boolean=w759) -> (0, 1=w766:i16)
            n564 = To Unsigned Word Integer(number=w766) -> (unsigned 16bit integer=w763:u16)
            n565 = feedback #52(u16 0) -> (w764:u16)
            n566 = Add(x=w763, y=w764) -> (x+y=w762:u16)
            "DIO Late Counter" <- w762
            n567 = feedback-in #52(w762) -> ()
            n568 = Subtract(x=w781, y=w760) -> (x-y=w780:u32)
            n569 = Split Number(x=w822) -> (hi(x)=w821:u32, lo(x)=w820:u32)
            n570 = Split Number(x=w811) -> (hi(x)=w816:u32, lo(x)=w815:u32)
            n571 = Boolean To (0,1)(Boolean="+ phase (DIO)") -> (0, 1=w777:i16)
            n572 = Split Number(x=w821) -> (lo(x)=w819:u16)  [unwired: 1 out]
            n573 = Split Number(x=w820) -> (hi(x)=w818:u16, lo(x)=w817:u16)
            n574 = Split Number(x=w816) -> (lo(x)=w814:u16)  [unwired: 1 out]
            n575 = Split Number(x=w815) -> (hi(x)=w813:u16, lo(x)=w812:u16)
            n576 = Split Number(x=w770) -> (hi(x)=w772:u8, lo(x)=w771:u8)
            n577 = Split Number(x=w767) -> (hi(x)=w769:u8, lo(x)=w768:u8)
            n578 = Split Number(x=w819) -> (hi(x)=w809:u8, lo(x)=w808:u8)
            n579 = Split Number(x=w818) -> (hi(x)=w807:u8, lo(x)=w806:u8)
            n580 = Split Number(x=w814) -> (hi(x)=w802:u8, lo(x)=w801:u8)
            n581 = Split Number(x=w817) -> (hi(x)=w805:u8, lo(x)=w804:u8)
            n582 = Split Number(x=w813) -> (hi(x)=w800:u8, lo(x)=w799:u8)
            n583 = Split Number(x=w812) -> (hi(x)=w798:u8, lo(x)=w797:u8)
            n584 = Multiply(x=w777, y="Phase count adjustment (DIO)") -> (x*y=w773:i16)
            n585 = feedback #53(i16 0) -> (w775:i16)
            n586 = Subtract(x=w775, y=w773) -> (x-y=w774:i16)
            "DIO Relative phase" <- w774
            n587 = feedback-in #53(w774) -> ()
            n588 = Add(x=w780, y=w773) -> (x+y=w779:u32)
            n589 = Build Array "BD 1 A Stack"(w772, w771) -> (w794:u8[])
            n590 = Build Array "BD 2 A Stack"(w769, w768) -> (w793:u8[])
            n591 = Build Array "BD 1 nu Stack"(w809, w808, w807, w806, w805, w804) -> (w803:u8[])
            n592 = Build Array "BD 2 nu Stack"(w802, w801, w800, w799, w798, w797) -> (w796:u8[])
            n593 = case shown="2" w810 {
              tunnel: [w860 w863] -> w792
              tunnel: [u8 10 u8 4] -> w795
              tunnel: "Swap F1 and F2" -> [w861 w863]
              frame 2 {
                # "F2"
                n594 = Not(x=w861) -> (.not. x?=w860:bool)
              }
              frame 1, Default {
                # "low chooses F1"
                # "F1"
              }
            }
            n595 = case "If FPGA is controlling (toggling) RF synth" shown="True" w791 {
              tunnel: w803 -> [_ w839]
              tunnel: w796 -> [_ w838]
              tunnel: w795 -> [_ w837]
              tunnel: w794 -> [_ w836]
              tunnel: w793 -> [_ w835]
              frame False {
              }
              frame True {
                # "Write next amp.\n(wait until beginning of next loop iteration to update)"
                n596 = flat-sequence "Update the next F1 and F2 frequency value (the actual frequency won't change until FSK is switched).\nThen load the next amplitude value into buffer, but don't update it until the next cycle." {
                  tunnel: w839 -> [w842]
                  tunnel: w838 -> [w841]
                  tunnel: w837 -> [w840]
                  tunnel: w836 -> [w853]
                  tunnel: w835 -> [w852]
                  frame #0 {
                    n597 = for {
                      tunnel: w842 -> [w848] mode=indexing
                      tunnel: w841 -> [w847] mode=indexing
                      tunnel: w840 -> [w845]
                      i -> [w846]
                      # "Write next freq."
                      n598 = To Unsigned Byte Integer(number=w846) -> (unsigned 8bit integer=w843:u8)
                      n599 = Add(x=w845, y=w843) -> (x+y=w844:u8)
                      n600 = call "write to RF synth bd.vi"("Address Byte"=w844, "BD 2 Byte"=w847, "BD 1 Byte"=w848) -> ()
                    }
                  }
                  frame #1 {
                    # "send udclk high"
                    n601 = xnode "FPGA I/O Node"("Connector1/DIO30"=TRUE ("Connector1/DIO15")) -> ()  [unwired: 1 in, 1 out]
                  }
                  frame #2 {
                    n602 = xnode "FPGA I/O Node"("Connector1/DIO30"=FALSE ("Connector1/DIO15")) -> ()  [unwired: 1 in, 1 out]
                  }
                  frame #3 {
                    n603 = for {
                      tunnel: w853 -> [w859] mode=indexing
                      tunnel: w852 -> [w858] mode=indexing
                      tunnel: u8 33 -> [w856]
                      i -> [w857]
                      n604 = To Unsigned Byte Integer(number=w857) -> (unsigned 8bit integer=w854:u8)
                      n605 = Add(x=w856, y=w854) -> (x+y=w855:u8)
                      n606 = call "write to RF synth bd.vi"("Address Byte"=w855, "BD 2 Byte"=w858, "BD 1 Byte"=w859) -> ()
                    }
                  }
                }
              }
            }
          }
        }
      }
    }
  }
  n607 = node-c288(w4) -> ()
  n608 = while "633 nm red excitation laser intensity feedback measurement" {
    shift-right: [w1072] -> _
    shift-left: w1 -> [w1077]
    stop <- FALSE stop-if-true
    n609 = flat-sequence {
      tunnel: w1077 -> [w1079]
      tunnel: [w1080] -> w1075
      tunnel: [w1079] -> w1073
      tunnel: [w1084] -> w1076
      tunnel: w1075 -> [w1084]
      tunnel: [w1083] -> w1074
      tunnel: w1073 -> [w1083]
      tunnel: [w1096] -> w1072
      tunnel: w1076 -> [w1107]
      tunnel: w1074 -> [w1104]
      frame #0 {
        n610 = call "Loop Timer12"("Count(Ticks)"=w1079) -> ("Tick Count(Ticks)"=w1080:u32)
      }
      frame #1 {
        n611 = xnode "FPGA I/O Node"("Connector1/DIO29"=TRUE ("Connector1/DIO35")) -> ("Chassis2/Mod1/AI2"=→"Red FB Intensity":i16)  [unwired: 2 in, 2 out]
      }
      frame #2 {
        n612 = feedback-in #54(w1107) -> ()
        n613 = feedback #54(w1107) -> (w1106:u32)
        n614 = Subtract(x=w1107, y=w1106) -> (x-y=w1105:u32)
        n615 = xnode "FPGA I/O Node"("Connector1/DIO29"=FALSE ("Connector1/DIO35")) -> ()  [unwired: 1 in, 1 out]
        n616 = Subtract(x=w1105, y=w1104) -> (x-y=w1086:u32)
        n617 = Subtract(x="Red FB Count", y=w1086) -> (x-y=w1100:u32)
        n618 = Number To Boolean Array(number=w1086) -> (Boolean array=w1087:bool[])
        n619 = Or Array Elements(Boolean array=w1087) -> (logical OR=w1085:bool)
        "Red FB Late?" <- w1085
        n620 = Boolean To (0,1)(Boolean="+ phase (Red FB)") -> (0, 1=w1098:i16)
        n621 = Boolean To (0,1)(Boolean=w1085) -> (0, 1=w1092:i16)
        n622 = Multiply(x=w1098, y="Phase count adjustment (Red FB)") -> (x*y=w1093:i16)
        n623 = Add(x=w1100, y=w1093) -> (x+y=w1096:u32)
        n624 = To Unsigned Word Integer(number=w1092) -> (unsigned 16bit integer=w1089:u16)
        n625 = feedback #55(i16 0) -> (w1095:i16)
        n626 = Subtract(x=w1095, y=w1093) -> (x-y=w1094:i16)
        "Red FB Relative Phase" <- w1094
        n627 = feedback-in #55(w1094) -> ()
        n628 = feedback #56(u16 0) -> (w1090:u16)
        n629 = Add(x=w1089, y=w1090) -> (x+y=w1088:u16)
        "Red Late Counter" <- w1088
        n630 = feedback-in #56(w1088) -> ()
      }
    }
  }
  n631 = while "633 nm red  fluorescent laser interlacing (DO to IA 633 nm AOM ME amp)." {
    shift-right: [w1111] -> _
    shift-left: w1 -> [w1116]
    shift-right: [w1110] -> _
    shift-left: _ -> [w1108]
    stop <- FALSE stop-if-true
    n632 = flat-sequence {
      tunnel: w1116 -> [w1119]
      tunnel: [w1120] -> w1114
      tunnel: [w1119] -> w1112
      tunnel: [w1118] -> w1109
      tunnel: w1108 -> [w1118]
      tunnel: [w1123] -> w1115
      tunnel: w1114 -> [w1123]
      tunnel: [w1122] -> w1113
      tunnel: w1112 -> [w1122]
      tunnel: w1109 -> [w1121]
      tunnel: [w1132] -> w1111
      tunnel: w1115 -> [w1152]
      tunnel: w1113 -> [w1149]
      tunnel: [w1141] -> w1110
      frame #0 {
        n633 = call "Loop Timer11"("Count(Ticks)"=w1119) -> ("Tick Count(Ticks)"=w1120:u32)
      }
      frame #1 {
        n634 = xnode "FPGA I/O Node"("Connector1/DIO32"=w1121, "Connector1/DIO33"=w1121, "Connector1/DIO34"=w1121) -> ()  [unwired: 3 in, 3 out]
      }
      frame #2 {
        n635 = feedback-in #57(w1152) -> ()
        n636 = feedback #57(w1152) -> (w1151:u32)
        n637 = Subtract(x=w1152, y=w1151) -> (x-y=w1150:u32)
        n638 = Subtract(x=w1150, y=w1149) -> (x-y=w1125:u32)
        n639 = Number To Boolean Array(number=w1125) -> (Boolean array=w1126:bool[])
        n640 = Or Array Elements(Boolean array=w1126) -> (logical OR=w1124:bool)
        "RI Late?" <- w1124
        n641 = Boolean To (0,1)(Boolean="+ phase (RI)") -> (0, 1=w1137:i16)
        n642 = Multiply(x=w1137, y="Phase count adjustment (RI)") -> (x*y=w1134:i16)
        n643 = Boolean To (0,1)(Boolean=w1124) -> (0, 1=w1131:i16)
        n644 = To Unsigned Word Integer(number=w1131) -> (unsigned 16bit integer=w1128:u16)
        n645 = feedback #58(i16 0) -> (w1135:i16)
        n646 = feedback #59(u16 0) -> (w1129:u16)
        n647 = Add(x=w1128, y=w1129) -> (x+y=w1127:u16)
        "RI Late Counter" <- w1127
        n648 = feedback-in #59(w1127) -> ()
        n649 = Subtract(x=w1135, y=w1134) -> (x-y=w1133:i16)
        "RI Relative phase" <- w1133
        n650 = feedback-in #58(w1133) -> ()
        n651 = feedback #60(TRUE) -> (w1144:bool)
        n652 = case shown="2" "Red Laser Operating Mode" {
          tunnel: [TRUE FALSE w1158] -> w1141
          tunnel: w1144 -> [_ _ w1155]
          frame 0, Default {
          }
          frame 1 {
          }
          frame 2 {
            n653 = Not(x=w1155) -> (.not. x?=w1157:bool)
            n654 = Select(t=w1157, s="Invert RI", f=w1155) -> (s? t:f=w1158:bool)
          }
        }
        n655 = Not(x=w1144) -> (.not. x?=w1140:bool)
        n656 = Select(t="Red interlace ON count", s=w1140, f="Red interlace OFF count") -> (s? t:f=w1146:u32)
        n657 = Subtract(x=w1146, y=w1125) -> (x-y=w1138:u32)
        n658 = Add(x=w1138, y=w1134) -> (x+y=w1132:u32)
        n659 = feedback-in #60(w1140) -> ()
      }
    }
  }
